vi "Intensity Measurement 2.0.vi"() -> ()   [LabVIEW 2012]
uses:
  <vilib>/Analysis/NI_AAL_SigProc.lvlib
  <vilib>/Analysis/NI_AALBase.lvlib
  <userlib>/_OpenG.lib/array/array.llb/Index 1D Array Elements (DBL)__ogtk.vi
  <vilib>/Analysis/baseanly.llb/Mean (DBL).vi
  Intensity Data.ctl
  <vilib>/Utility/file.llb/Read From Spreadsheet File (I64).vi
  <vilib>/Utility/miscctls.llb/LVPointTypeDef.ctl
  <userlib>/_OpenG.lib/array/array.llb/Conditional Auto-Indexing Tunnel (DBL)__ogtk.vi
  <userlib>/_OpenG.lib/array/array.llb/Conditional Auto-Indexing Tunnel (U32)__ogtk.vi
  <userlib>/_OpenG.lib/array/array.llb/Index 1D Array Elements (U32)__ogtk.vi
  <vilib>/Analysis/6fits.llb/Curve Fitting Criteria.ctl
  <vilib>/Analysis/NI_AALPro.lvlib
panel:
  in  "Tab Control":enum32{"Normalization", "Fitting", "Statistics"}(tab)
  out "Normalization Curve":dbl[](graph)
  out "Normalization Selections":cluster{i32[], i32[]}(graph)
  in  "Reset Normalization Cursors":bool
  in  "Array Type":bool=TRUE
  in  "Load New Data":bool
  in  "pixels/um":dbl=1.0
  in  "Previous Cell":bool
  in  "Next Cell":bool
  in  "Gaussian Fit Method":T1 items=["Least Square", "Least Absolute Residual", "Bisquare"]
  out "Normalized Intensity Maximums":T2(graph)
  out "FWHM":dbl
  out "center":dbl
  out "residue":dbl
  out "amplitude":dbl
  out "Selected Frame":dbl
  out "Peak Fitting":cluster{"Locations":dbl[], "Amplitudes":dbl[]}[](graph)
  in  "Intensity Threshold":i32=50
  out "Cells Identified":i32
  in  "Padding":u32=3
  in  "Target Baseline (%)":dbl=10.0
  out "Cell Width Histogram":T3(graph)
  in  "location histogram interval":i32=10 caption="histogram interval"
  out "Cell Location histogram":T3(graph)
  in  "Gate Width":u32=8 caption="um"
  in  "Gate Center":u32=10 caption="um"
  out "% population\nin gate":dbl
  in  "find best gate center":bool
  out "Arrival time delta histogram":T3(graph)
  in  "Frame Rate":u32=1 min=1 step=1
  in  "arrival histogram interval":i32=10 caption="histogram interval"
  in  "delta threshold":dbl min=0.0
  out "Cell Count":i32
  in  "cell width histo intervals":i32=10 caption="histogram interval"
  # "Cell Selector"
  # "Gaussian Fit"
  # "Statistics"
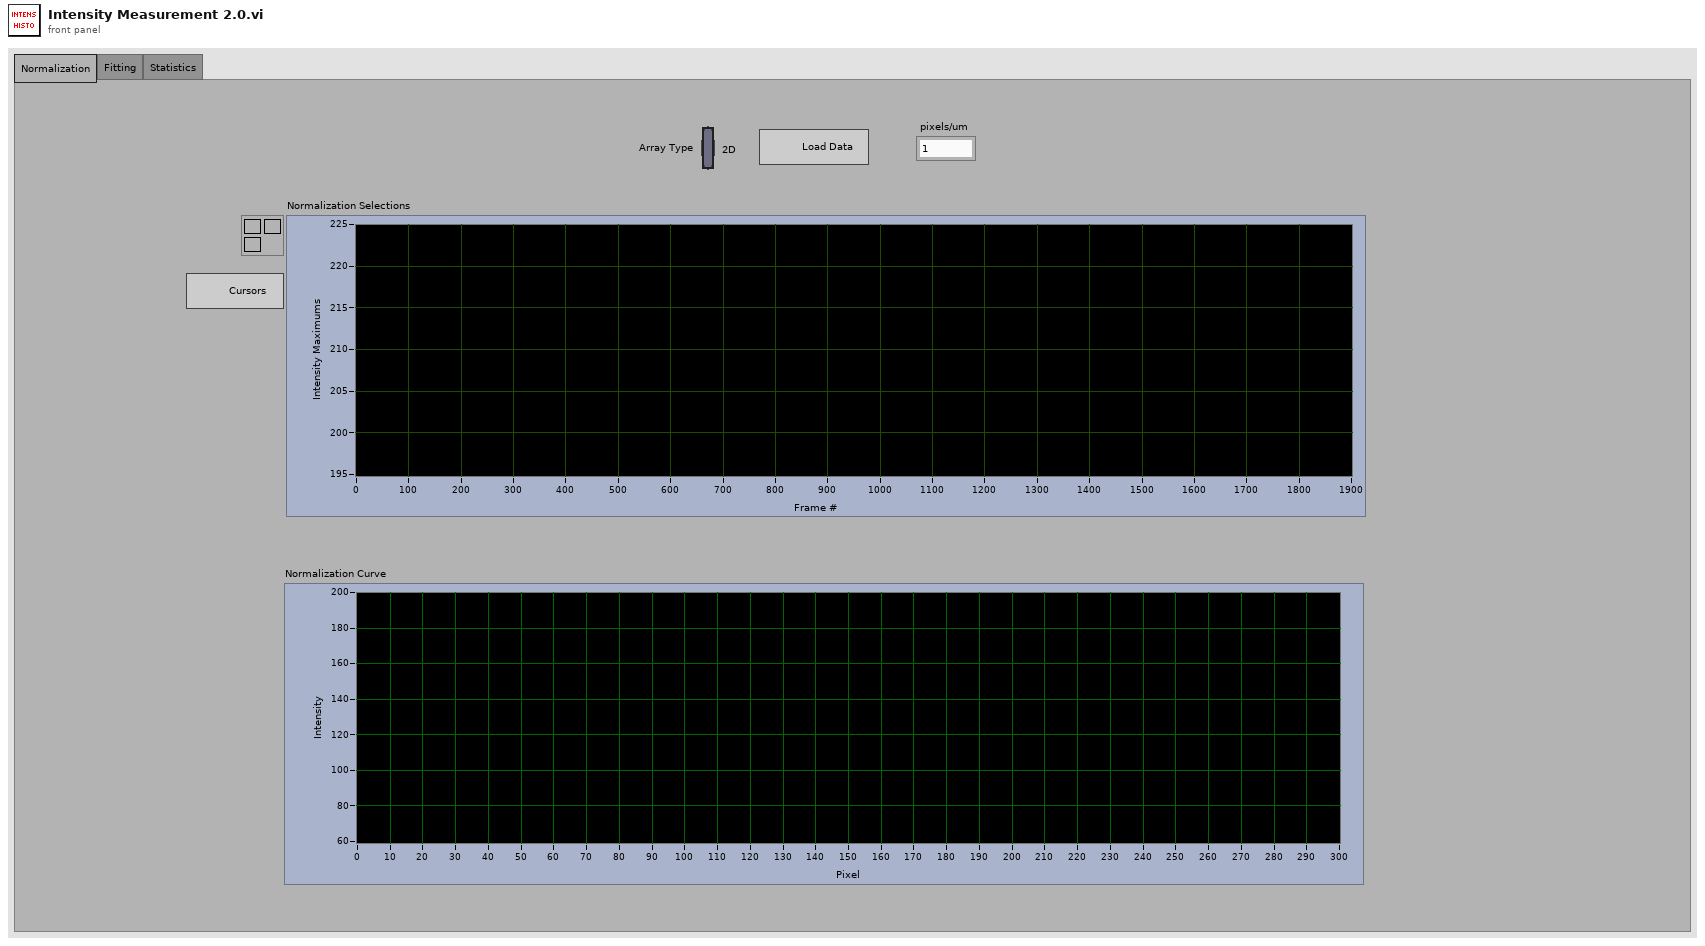
[diagram p1: front panel]
types:
  T1 = typedef "NI_AALPro.lvlib/Curve Fitting Criteria.ctl" = u16
  T2 = cluster{"Cell Location (frame)":u32[], "Cell Amplitude":dbl[]}[]
  T3 = cluster{"X Values":dbl[], "Histogram: h(x)":i32[]}
  T4 = enum32{"invalid app kind", "Development System", "Run Time System", "Student Edition", "Embedded LabVIEW", "Evaluation", "Custom"}
  T5 = cluster{"peak location (frame)":u32[], "Peak Amplitude":dbl[]}[]
  T6 = typedef "LVPointTypeDef.ctl" = cluster{"Horizontal":i16, "Vertical":i16}
  T7 = enum32{"Invalid", "Standard", "Closed", "Hidden", "Minimized", "Maximized"}
  T8 = typedef "Intensity Data.ctl" = cluster{"Raw Data":i32[][], "Normalized Intensity Data":dbl[][], "Frame Count":u32, "Pixel Count":u32, "Interrogation Width (um)":dbl, "Fitting Range":u32[], "Frame Indexed":cluster{"intensity peak":dbl[], "peak location (um)":dbl[]}, "Cell Indexed":cluster{"Cell Location (frame)":u32[], "Cell Amplitude":dbl[], "Cell Location (um)":dbl[], "Cell Width (um)":dbl[], "Cell Arrival Delta (frame)":dbl[], "Cell Arrival Delta (us)":dbl[]}}
  T9 = cluster{"Core":cluster{"Current VI Reference":refnum<vi>, "Close Panel on Exit?":bool}, "Intensity Data Location":path, "pixels/um":dbl, "Intensity Data":T8, "Gated Data":cluster{"Gate Width":u32, "Gate Center":u32, "Cell Indexed":cluster{"Peak Amplitude":dbl[], "peak location (frame)":u32[], "peak location (um)":dbl[]}}}
  T10 = typedef "LVRangeTypeDef.ctl" = cluster{"Minimum":dbl, "Maximum":dbl, "Increment":dbl, "Minor Increment":dbl, "Start":dbl}
  T11 = typedef "LVCursorListTypeDef.ctl" = cluster{"Name":string, "Color":u32, "Style":u8, "Point Style":u8, "Name Visible":bool, "Allow Drag":bool, "Cursor Mode":u32, "Plot":i32, "Index":i32, "Position":cluster{"X":dbl, "Y":dbl}, "X Scale":u32, "Y Scale":u32, "Watch Plots":i32[], "Watch All Plots":bool, "Plot Area":i32, "Label Offset":cluster{"X":dbl, "Y":dbl}}[]
  T12 = cluster{"Name":string, "Color":u32, "Style":u8, "Point Style":u8, "Name Visible":bool, "Allow Drag":bool, "Cursor Mode":u32, "Plot":i32, "Index":i32, "Position":cluster{"X":dbl, "Y":dbl}, "X Scale":u32, "Y Scale":u32, "Watch Plots":i32[], "Watch All Plots":bool, "Plot Area":i32, "Label Offset":cluster{"X":dbl, "Y":dbl}}
  T13 = cluster{"Name":string, "Color":u32, "Style":u8, "Point Style":u8, "Name Visible":bool, "Allow Drag":bool, "Cursor Mode":u32, "Plot":i32, "Index":i32, "Position":cluster{"X":dbl, "Y":dbl}, "X Scale":u32, "Y Scale":u32, "Watch Plots":i32[], "Watch All Plots":bool, "Plot Area":i32, "Label Offset":cluster{"X":dbl, "Y":dbl}}[]
  T14 = cluster{"Gate Width":u32, "Gate Center":u32, "Cell Indexed":cluster{"Peak Amplitude":dbl[], "peak location (frame)":u32[], "peak location (um)":dbl[]}}
  T15 = cluster{"Current VI Reference":refnum<vi>, "Close Panel on Exit?":bool}
  T16 = cluster{"amplitude":dbl, "center":dbl, "FWHM":dbl, "residue":dbl, "Best Gaussian Fit":dbl[]}
  T17 = cluster{"Cell Location (frame)":u32[], "Cell Amplitude":dbl[]}
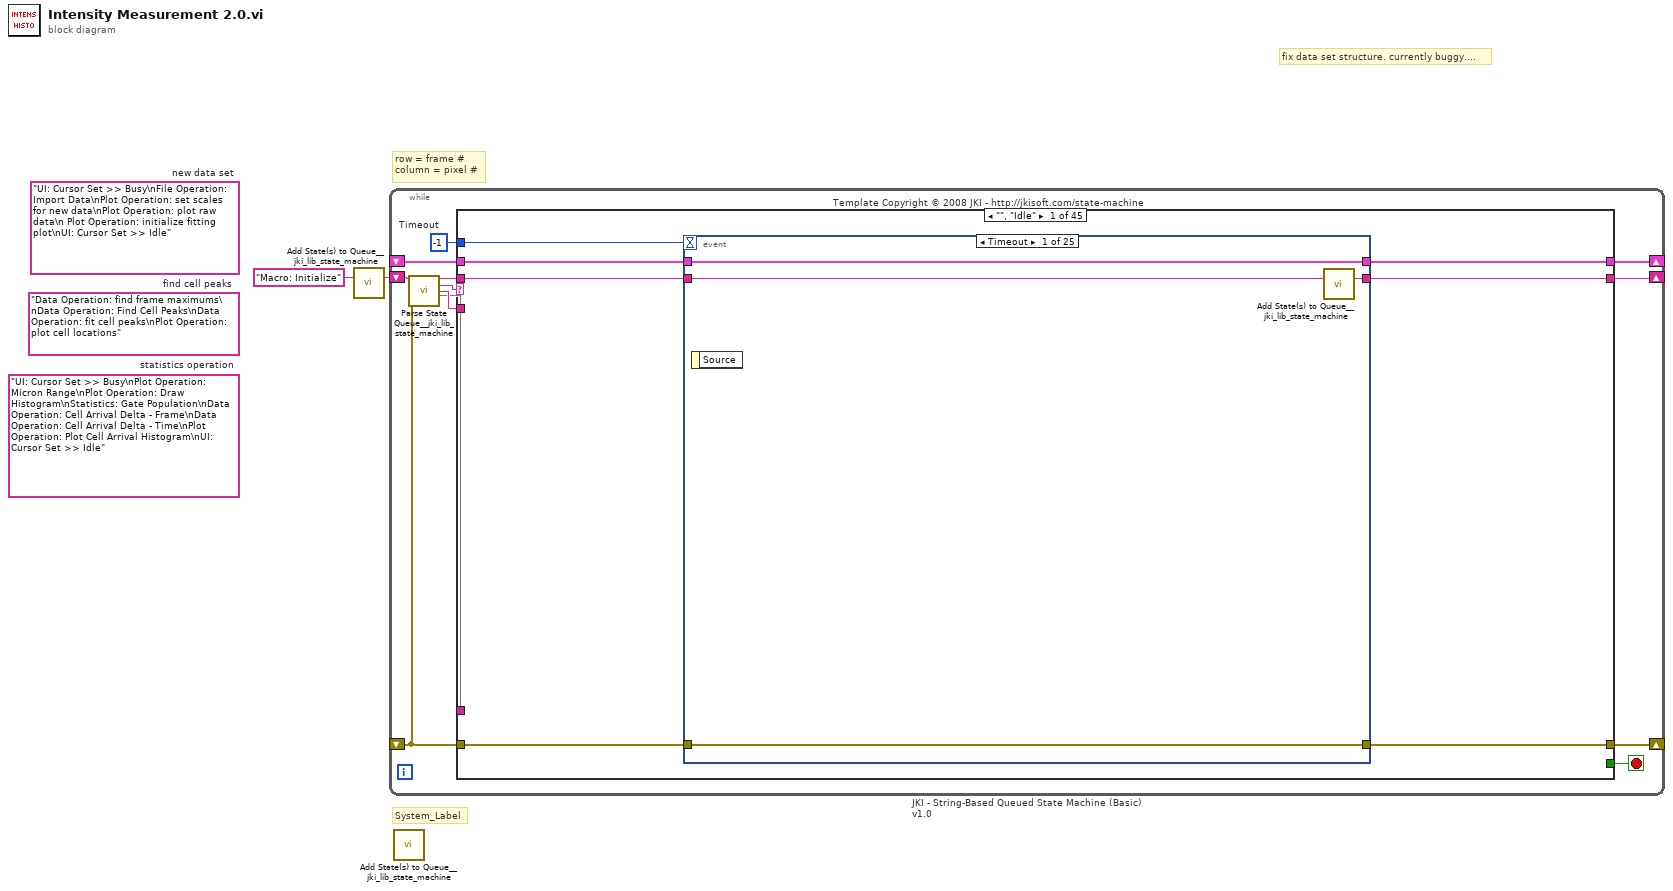
[diagram p0: block diagram]
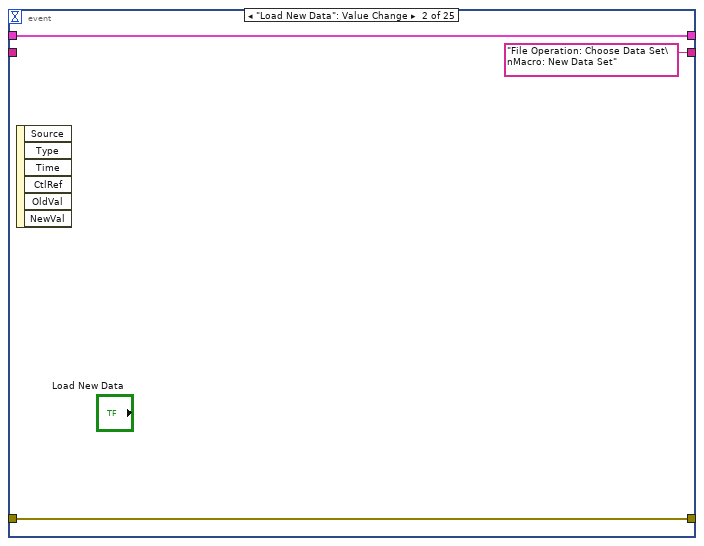
[diagram p2: hidden frame]
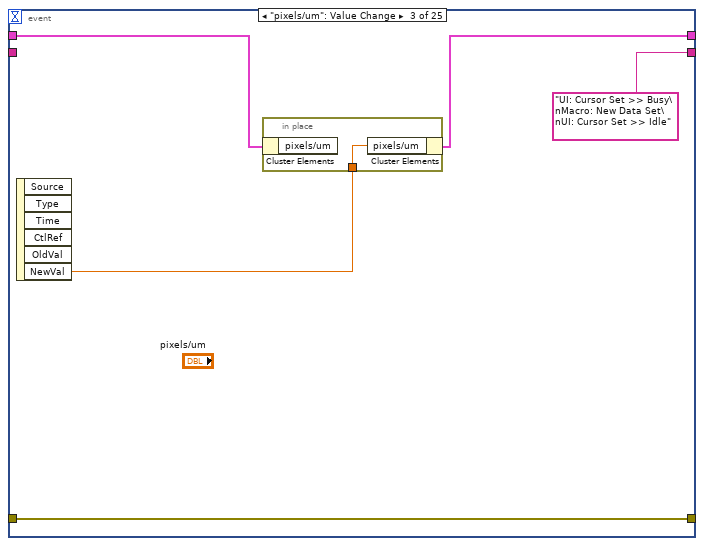
[diagram p3: hidden frame]
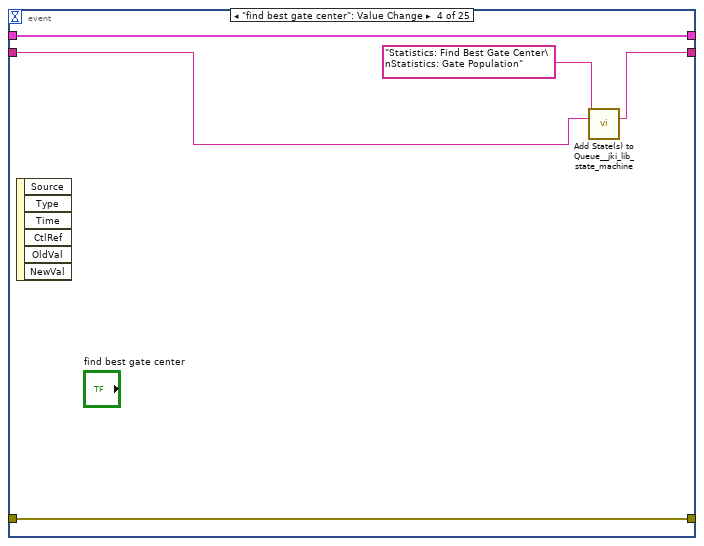
[diagram p4: hidden frame]
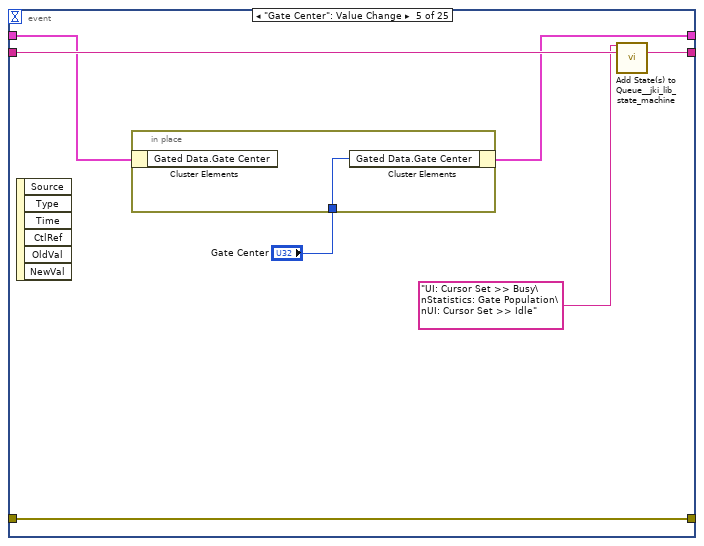
[diagram p5: hidden frame]
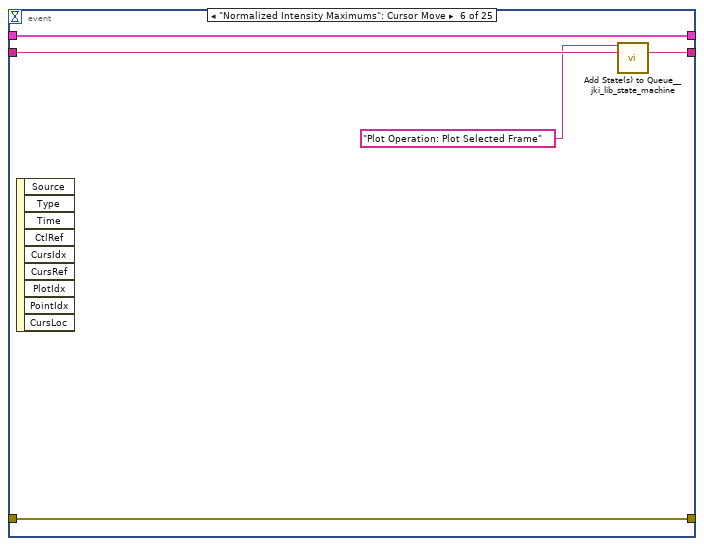
[diagram p6: hidden frame]
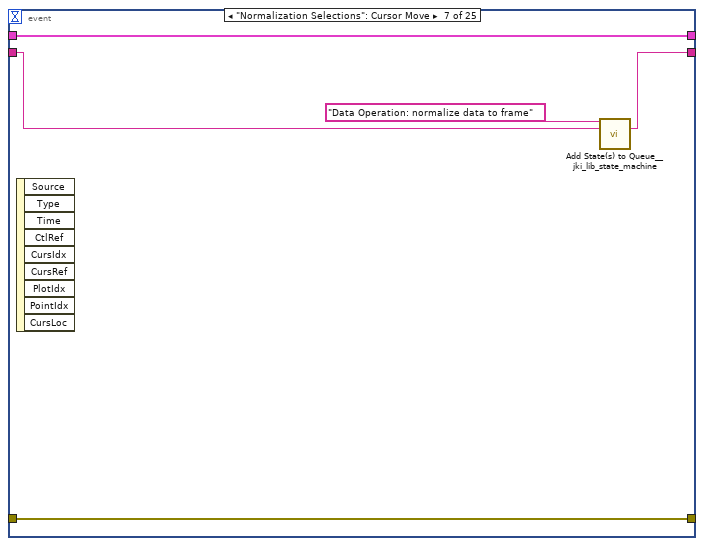
[diagram p7: hidden frame]
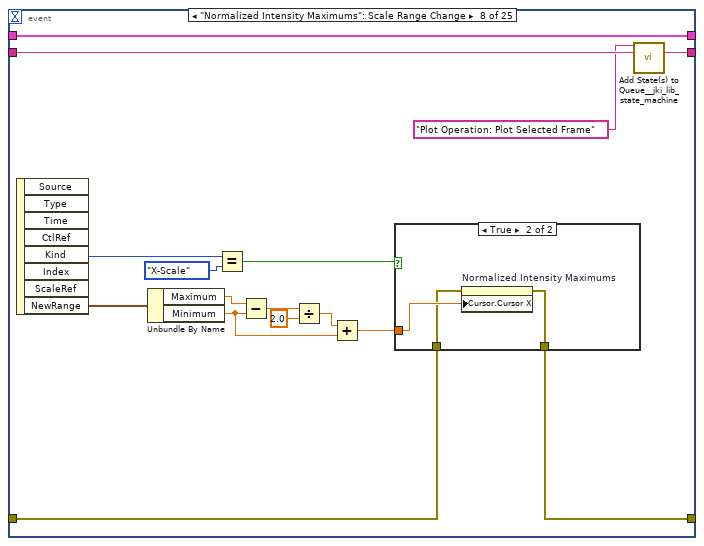
[diagram p8: hidden frame]
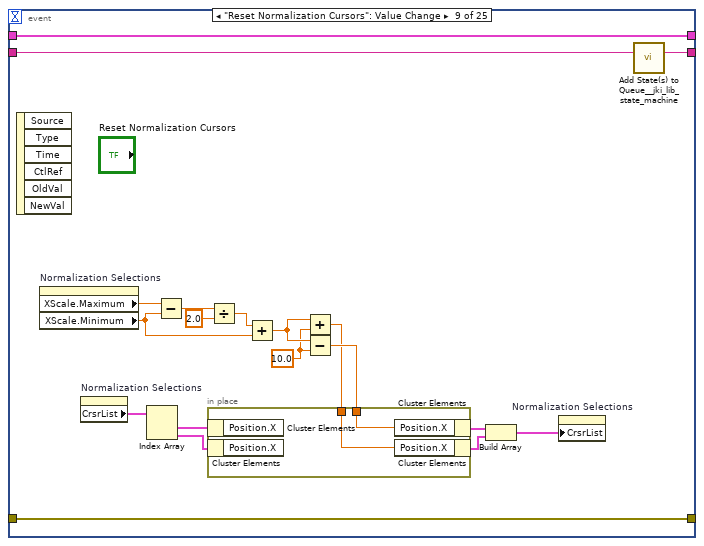
[diagram p10: hidden frame]
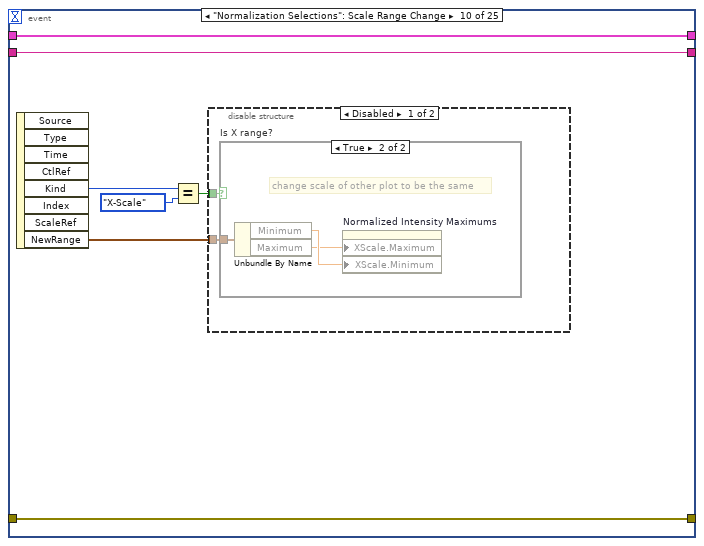
[diagram p11: hidden frame]
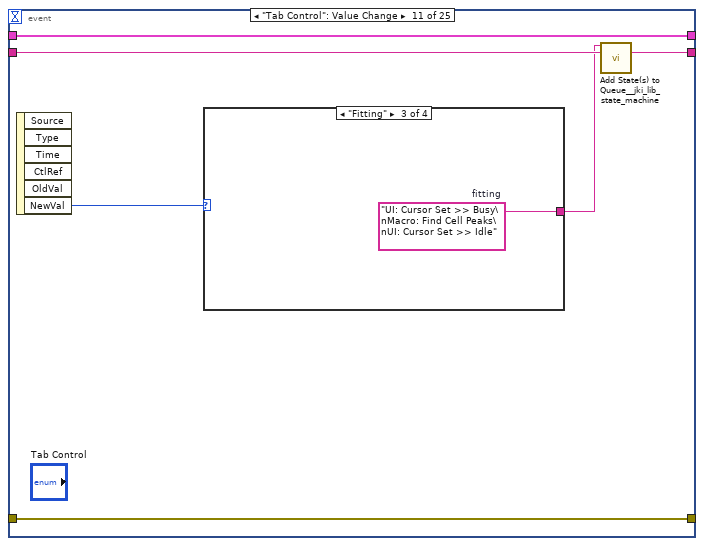
[diagram p14: hidden frame]
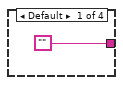
[diagram p15: hidden frame]
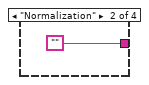
[diagram p16: hidden frame]
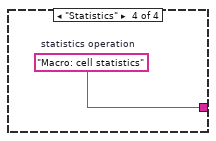
[diagram p17: hidden frame]
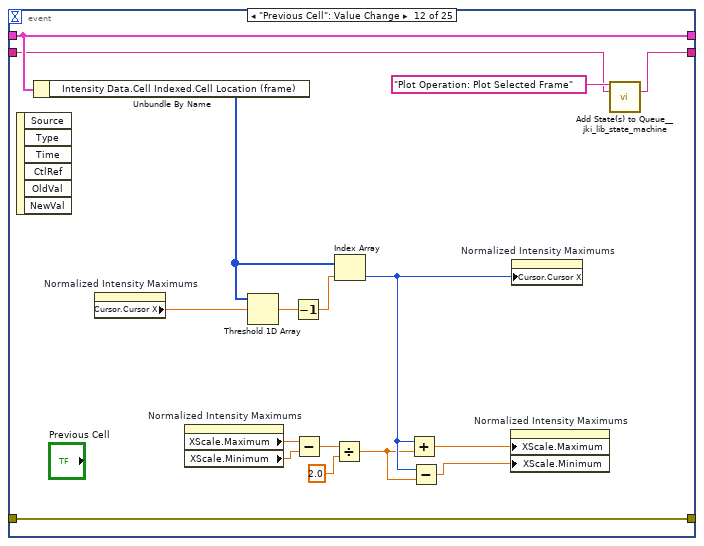
[diagram p18: hidden frame]
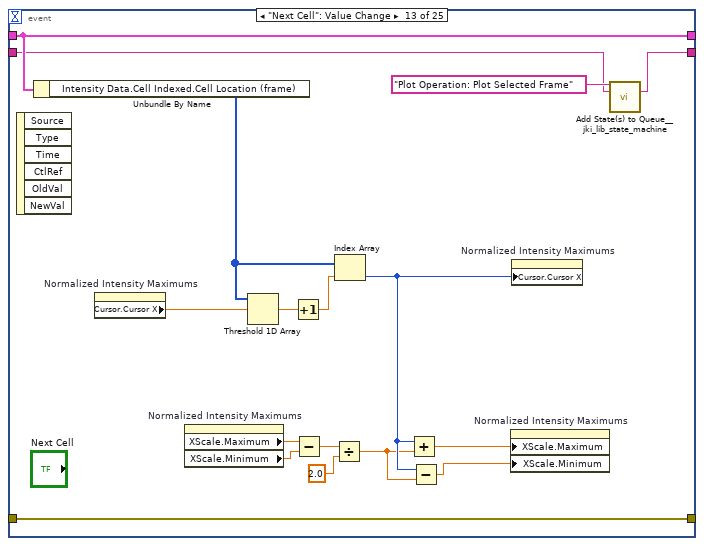
[diagram p19: hidden frame]
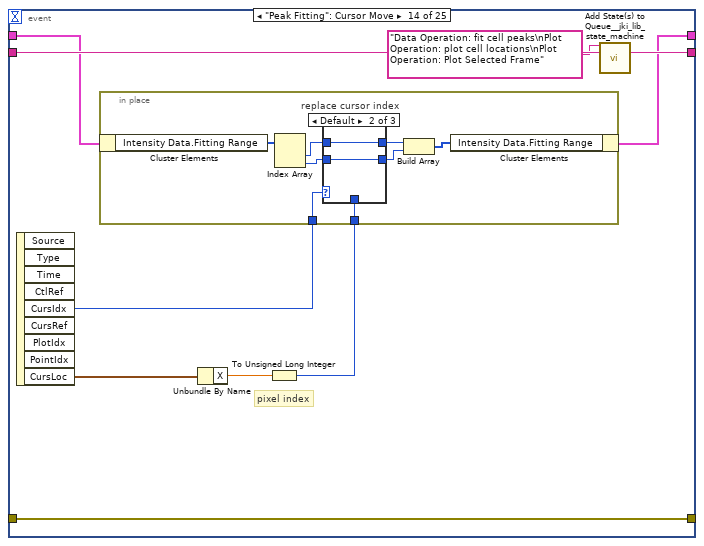
[diagram p20: hidden frame]
diagram:
  (unwired) "UI: Cursor Set >> Busy\nFile Operation: Import Data\nPlot Operation: set scales for new data\nPlot Operation: plot raw data\n Plot Operation: initialize fitting plot\nUI: Cursor Set >> Idle"  # new data set
  (unwired) "Data Operation: find frame maximums\nData Operation: Find Cell Peaks\nData Operation: fit cell peaks\nPlot Operation: plot cell locations"  # find cell peaks
  (unwired) "UI: Cursor Set >> Busy\nPlot Operation: Micron Range\nPlot Operation: Draw Histogram\nStatistics: Gate Population\nData Operation: Cell Arrival Delta - Frame\nData Operation: Cell Arrival Delta - Time\nPlot Operation: Plot Cell Arrival Histogram\nUI: Cursor Set >> Idle"  # statistics operation
  # "fix data set structure. currently buggy...."
  # "row = frame #\ncolumn = pixel #"
  # "System_Label"
  n1 = call <vilib>:"Add State(s) to Queue__jki_lib_state_machine.vi"("State(s) in (\"\")"="Macro: Initialize") -> ("States Out"=w2:string)  [unwired: 14 in]
  n2 = while "JKI - String-Based Queued State Machine (Basic) v1.0" {
    shift-right: [w7] -> _
    shift-left: _ -> [w6]
    shift-right: [w10] -> _
    shift-left: _ -> [w4]
    shift-right: [w9] -> _
    shift-left: w2 -> [w11]
    stop <- w8 stop-if-true
    w5 = -1  # Timeout
    # "Template Copyright © 2008 JKI - http://jkisoft.com/state-machine"
    n3 = call <vilib>:"Parse State Queue__jki_lib_state_machine.vi"("State Queue"=w11, "Error In (no error)"=w4) -> ("Remaining States"=w13:string, "Current State"=w14:string, "Arguments"=w12:string, 14:w3)  [unwired: 10 in]
    n4 = case shown="\"\", \"Idle\"" w14 {
      selector: w14 -> [_ _ w240 _ _ _ _ _ _ _ _ _ _ _ _ _ _ _ _ _ _ _ _ _ _ _ _ _ _ _ _ _ _ _ _ _ _ _ _ _ _ _ _ _ _]
      tunnel: w13 -> [w21 w239 w244 w262 _ w277 w281 w293 w299 w303 w314 w333 w339 w350 w376 w381 w386 w391 w396 w406 w410 w428 w451 w471 w486 w515 w542 w553 w573 w578 w585 w595 w615 w631 w647 w663 w681 w692 w701 w706 w726 w742 w751 w757 w790]
      tunnel: w12 -> [_ _ _ _ _ _ _ _ _ _ _ _ w334 w344 _ _ _ _ _ _ _ _ _ _ _ _ _ _ _ _ _ _ _ _ _ _ _ _ _ _ _ _ _ _ _]
      tunnel: w6 -> [w19 w236 w242 w253 w267 w275 w278 _ w294 w300 w311 w322 w337 w346 w373 w378 w383 w388 w393 w403 w407 w425 w446 w468 w482 w512 w539 w548 w567 w575 w582 w597 w612 w629 w636 w661 w679 w688 w698 w703 w724 w732 w748 w759 w785]
      tunnel: [w18 w237 w246 w259 errorcluster {"status"=FALSE, "code"=0, "source"=""} ("error out") w274 w279 w290 w295 w301 w312 w325 w335 w347 w374 w379 w384 w389 w394 w404 w408 w429 w447 w465 w478 w506 w540 w551 w571 w576 w583 w593 w613 w621 w645 w656 w667 w685 w694 w704 w711 w740 w749 w760 w786] -> w10
      tunnel: w4 -> [w17 w237 w245 w259 w265 w274 w279 w290 w296 w301 w312 w324 w336 w348 w374 w379 w384 w389 w394 w404 w408 w420 w448 w465 w480 w507 w540 w551 w571 w576 w583 w596 w613 w621 w645 w657 w678 w686 w702 w704 w712 w740 w749 w761 w787]
      tunnel: [w20 w238 w243 w261 "UI: Cursor Set >> Idle" ("States Out") w276 w280 w292 w298 w302 w313 w332 w338 w349 w375 w380 w385 w390 w395 w405 w409 w427 w450 w470 w485 w514 w541 w552 w572 w577 w584 w594 w614 w630 w646 w662 w680 w691 w700 w705 w725 w741 w750 w756 w789] -> w9
      tunnel: [_ _ _ _ _ TRUE _ _ _ _ _ _ _ _ _ _ _ _ _ _ _ _ _ _ _ _ _ _ _ _ _ _ _ _ _ _ _ _ _ _ _ _ _ _ _] -> w8
      tunnel: [w16 w236 w242 w260 w267 w275 w278 w291 w294 w300 w311 w322 w337 w346 w373 w378 w383 w388 w393 w403 w407 w426 w445 w467 w479 w510 w538 w547 w566 w575 w582 w597 w612 w629 w637 w661 w679 w688 w698 w703 w723 w731 w748 w758 w784] -> w7
      tunnel: w5 -> [w15 _ _ _ _ _ _ _ _ _ _ _ _ _ _ _ _ _ _ _ _ _ _ _ _ _ _ _ _ _ _ _ _ _ _ _ _ _ _ _ _ _ _ _ _]
      tunnel: w3 -> [_ _ _ _ w263 _ _ _ _ _ _ _ _ _ _ _ _ _ _ _ _ _ _ _ _ _ _ _ _ _ _ _ _ _ _ _ _ _ _ _ _ _ _ _ _]
      frame "", "Idle" {
        n5 = event shown="[0] Timeout" {
          selector: _ -> [_ _ _ _ _ _ _ _ _ _ _ _ _ _ _ _ _ _ _ _ _ _ _ _ _]
          dyn-events: _ -> [_ _ _ _ _ _ _ _ _ _ _ _ _ _ _ _ _ _ _ _ _ _ _ _ _]
          timeout: w15 -> [_ _ _ _ _ _ _ _ _ _ _ _ _ _ _ _ _ _ _ _ _ _ _ _ _]
          tunnel: w21 -> [w25 _ _ w35 w44 w49 w55 w59 w91 w103 w113 w130 w147 w162 w180 w188 _ w197 w201 w206 w212 w216 w222 w225 w235]
          tunnel: [w24 "File Operation: Choose Data Set\nMacro: New Data Set" ("States Out") "UI: Cursor Set >> Busy\nMacro: New Data Set\nUI: Cursor Set >> Idle" ("States Out") w37 w45 w50 w53 w60 w92 w103 w112 w129 w146 w161 w179 w189 "UI: Cursor Set >> Busy\nPlot Operation: Draw Histogram\nUI: Cursor Set >> Idle" ("States Out") w196 w200 w207 w211 w215 w220 w226 w234] -> w20
          tunnel: w19 -> [w22 w28 w31 w38 w42 w51 w56 w73 w96 w104 w115 w136 w153 w160 w182 w186 w193 w198 w203 w208 w213 w218 w223 w228 w232]
          tunnel: [w23 w26 w32 w39 w46 w52 w57 w64 w85 w105 w116 w137 w154 w164 w183 w190 w194 w199 w204 w209 w214 w219 w224 w229 w233] -> w18
          tunnel: w17 -> [w23 w26 w32 w39 w46 w52 w57 w65 w85 w105 w116 w137 w154 w164 w183 w190 w194 w199 w204 w209 w214 w219 w224 w229 w233]
          tunnel: [w22 w28 w29 w38 w40 w51 w56 w73 w96 w104 w115 w136 w153 w159 w182 w185 w193 w198 w203 w208 w213 w218 w223 w228 w232] -> w16
          event Timeout {
            n6 = event-data() -> ()  [unwired: 1 in, 1 out]
            n7 = call <vilib>:"Add State(s) to Queue__jki_lib_state_machine.vi"("State(s) in (\"\")"=w25) -> ("States Out"=w24:string)  [unwired: 14 in]
          }
          event "Load New Data": Value Change {
            n8 = event-data() -> ()  [unwired: 1 in, 6 out]
          }
          event "pixels/um": Value Change {
            n9 = event-data() -> ("NewVal"=w30:dbl)  [unwired: 1 in, 5 out]
            n10 = in-place {
              in-place-border: w30 -> [w34]
              n11 = in-place-cluster #1(w31) -> ()  [unwired: 1 out]
              n12 = in-place-cluster #1("pixels/um"=w34) -> (w29:T9)
            }
          }
          event "find best gate center": Value Change {
            n13 = event-data() -> ()  [unwired: 1 in, 6 out]
            n14 = call <vilib>:"Add State(s) to Queue__jki_lib_state_machine.vi"("State(s) in Front (\"\")"="Statistics: Find Best Gate Center\nStatistics: Gate Population" ("State(s) in Front (\"\")"), "State(s) in (\"\")"=w35) -> ("States Out"=w37:string)  [unwired: 13 in]
          }
          event "Gate Center": Value Change {
            n15 = event-data() -> ()  [unwired: 1 in, 6 out]
            n16 = in-place {
              in-place-border: "Gate Center" -> [w47]
              n17 = in-place-cluster #2(w42) -> ()  [unwired: 1 out]
              n18 = in-place-cluster #2("Gated Data.Gate Center"=w47) -> (w40:T9)
            }
            n19 = call <vilib>:"Add State(s) to Queue__jki_lib_state_machine.vi"("State(s) in Front (\"\")"="UI: Cursor Set >> Busy\nStatistics: Gate Population\nUI: Cursor Set >> Idle" ("State(s) in Front (\"\")"), "State(s) in (\"\")"=w44) -> ("States Out"=w45:string)  [unwired: 13 in]
          }
          event "Normalized Intensity Maximums": Cursor Move {
            n20 = event-data() -> ()  [unwired: 1 in, 9 out]
            n21 = call <vilib>:"Add State(s) to Queue__jki_lib_state_machine.vi"("State(s) in Front (\"\")"="Plot Operation: Plot Selected Frame" ("State(s) in Front (\"\")"), "State(s) in (\"\")"=w49) -> ("States Out"=w50:string)  [unwired: 13 in]
          }
          event "Normalization Selections": Cursor Move {
            n22 = event-data() -> ()  [unwired: 1 in, 9 out]
            n23 = call <vilib>:"Add State(s) to Queue__jki_lib_state_machine.vi"("State(s) in Front (\"\")"="Data Operation: normalize data to frame" ("State(s) in Front (\"\")"), "State(s) in (\"\")"=w55) -> ("States Out"=w53:string)  [unwired: 13 in]
          }
          event "Normalized Intensity Maximums": Scale Range Change {
            n24 = event-data() -> ("Kind"=w72:enum16{"X-Scale", "Y-Scale", "Z-Scale"}, "NewRange"=w69:T10)  [unwired: 1 in, 6 out]
            n25 = Unbundle By Name(w69) -> ("Maximum"=w68:dbl, "Minimum"=w62:dbl)
            n26 = Equal?(x=w72, y=enum16{"X-Scale", "Y-Scale", "Z-Scale"}."X-Scale" ("Kind")) -> (x = y?=w70:bool)
            n27 = Subtract(x=w68, y=w62) -> (x-y=w67:dbl)
            n28 = Divide(x=w67, y=2.0) -> (x/y=w63:dbl)
            n29 = Add(x=w63, y=w62) -> (x+y=w61:dbl)
            n30 = case shown="True" w70 {
              tunnel: w61 -> [_ w77]
              tunnel: w65 -> [w74 w76]
              tunnel: [w74 w75] -> w64
              frame False {
              }
              frame True {
                n31 = property on="Normalized Intensity Maximums" class="XYGraph (strict)"(error in=w76, "Cursor.Cursor X"=w77) -> (error out=w75:errorcluster)  [unwired: 1 in, 1 out]
              }
            }
            n32 = call <vilib>:"Add State(s) to Queue__jki_lib_state_machine.vi"("State(s) in Front (\"\")"="Plot Operation: Plot Selected Frame" ("State(s) in Front (\"\")"), "State(s) in (\"\")"=w59) -> ("States Out"=w60:string)  [unwired: 13 in]
          }
          event "Reset Normalization Cursors": Value Change {
            w83 = 10.0 ("y")
            n33 = event-data() -> ()  [unwired: 1 in, 6 out]
            n34 = property on="Normalization Selections" class="XYGraph (strict)"() -> ("XScale.Maximum"=w87:dbl, "XScale.Minimum"=w86:dbl)  [unwired: 2 in, 2 out]
            n35 = property on="Normalization Selections" class="XYGraph (strict)"() -> ("CrsrList"=w90:T11)  [unwired: 2 in, 2 out]
            n36 = Index Array(array=w90) -> (element #1=w89:T12, element #2=w88:T12)  [unwired: 2 in]
            n37 = Subtract(x=w87, y=w86) -> (x-y=w95:dbl)
            n38 = Divide(x=w95, y=2.0) -> (x/y=w93:dbl)
            n39 = Add(x=w93, y=w86) -> (x+y=w84:dbl)
            n40 = Add(x=w84, y=w83) -> (x+y=w81:dbl)
            n41 = Subtract(x=w84, y=w83) -> (x-y=w82:dbl)
            n42 = in-place {
              in-place-border: w82 -> [w98]
              in-place-border: w81 -> [w97]
              n43 = in-place-cluster #3(w89) -> ()  [unwired: 1 out]
              n44 = in-place-cluster #4(w88) -> ()  [unwired: 1 out]
              n45 = in-place-cluster #3("Position.X"=w98) -> (w80:T12)
              n46 = in-place-cluster #4("Position.X"=w97) -> (w79:T12)
            }
            n47 = Build Array(w80, w79) -> (w78:T13)
            n48 = property on="Normalization Selections" class="XYGraph (strict)"("CrsrList"=w78) -> ()  [unwired: 2 in, 2 out]
            n49 = call <vilib>:"Add State(s) to Queue__jki_lib_state_machine.vi"("State(s) in (\"\")"=w91) -> ("States Out"=w92:string)  [unwired: 14 in]
          }
          event "Normalization Selections": Scale Range Change {
            n50 = event-data() -> ("Kind"=w100:enum16{"X-Scale", "Y-Scale", "Z-Scale"}, "NewRange"=w102:T10)  [unwired: 1 in, 6 out]
            n51 = Equal?(x=w100, y=enum16{"X-Scale", "Y-Scale", "Z-Scale"}."X-Scale" ("Kind")) -> (x = y?=w99:bool)
            n52 = disable-structure shown="Disabled" {
              disable-tunnel: w102 -> [w107 _]
              disable-tunnel: w99 -> [w106 _]
              frame Disabled {
                n53 = case "Is X range?" shown="True" w106 {
                  tunnel: w107 -> [_ w110]
                  frame False {
                  }
                  frame True {
                    # "change scale of other plot to be the same"
                    n54 = Unbundle By Name(w110) -> ("Minimum"=w109:dbl, "Maximum"=w108:dbl)
                    n55 = property on="Normalized Intensity Maximums" class="XYGraph (strict)"("XScale.Maximum"=w108, "XScale.Minimum"=w109) -> ()  [unwired: 2 in, 2 out]
                  }
                }
              }
              frame Enabled {
              }
            }
          }
          event "Tab Control": Value Change {
            n56 = event-data() -> ("NewVal"=w114:enum32{"Normalization", "Fitting", "Statistics"})  [unwired: 1 in, 5 out]
            n57 = case shown="\"Fitting\"" w114 {
              tunnel: ["" "" w119 w120] -> w111
              frame Default {
              }
              frame "Normalization" {
              }
              frame "Fitting" {
                w119 = "UI: Cursor Set >> Busy\nMacro: Find Cell Peaks\nUI: Cursor Set >> Idle"  # fitting
              }
              frame "Statistics" {
                w120 = "Macro: cell statistics"  # statistics operation
              }
            }
            n58 = call <vilib>:"Add State(s) to Queue__jki_lib_state_machine.vi"("State(s) in Front (\"\")"=w111, "State(s) in (\"\")"=w113) -> ("States Out"=w112:string)  [unwired: 13 in]
          }
          event "Previous Cell": Value Change {
            n59 = event-data() -> ()  [unwired: 1 in, 6 out]
            n60 = Unbundle By Name(w136) -> ("Intensity Data.Cell Indexed.Cell Location (frame)"=w134:u32[])
            n61 = property on="Normalized Intensity Maximums" class="XYGraph (strict)"() -> ("Cursor.Cursor X"=w135:dbl)  [unwired: 2 in, 2 out]
            n62 = property on="Normalized Intensity Maximums" class="XYGraph (strict)"() -> ("XScale.Maximum"=w128:dbl, "XScale.Minimum"=w127:dbl)  [unwired: 2 in, 2 out]
            n63 = Threshold 1D Array(2:w135, 3:w134) -> (0:w133:dbl)  [unwired: 1 in]
            n64 = Decrement(x=w133) -> (x-1=w132:dbl)
            n65 = Subtract(x=w128, y=w127) -> (x-y=w126:dbl)
            n66 = Divide(x=w126, y=2.0) -> (x/y=w123:dbl)
            n67 = Index Array(array=w134, index=w132) -> (element=w124:u32)
            n68 = Add(x=w124, y=w123) -> (x+y=w122:dbl)
            n69 = Subtract(x=w124, y=w123) -> (x-y=w121:dbl)
            n70 = property on="Normalized Intensity Maximums" class="XYGraph (strict)"("XScale.Maximum"=w122, "XScale.Minimum"=w121) -> ()  [unwired: 2 in, 2 out]
            n71 = property on="Normalized Intensity Maximums" class="XYGraph (strict)"("Cursor.Cursor X"=w124) -> ()  [unwired: 2 in, 2 out]
            n72 = call <vilib>:"Add State(s) to Queue__jki_lib_state_machine.vi"("State(s) in Front (\"\")"="Plot Operation: Plot Selected Frame" ("State(s) in Front (\"\")"), "State(s) in (\"\")"=w130) -> ("States Out"=w129:string)  [unwired: 13 in]
          }
          event "Next Cell": Value Change {
            n73 = event-data() -> ()  [unwired: 1 in, 6 out]
            n74 = Unbundle By Name(w153) -> ("Intensity Data.Cell Indexed.Cell Location (frame)"=w151:u32[])
            n75 = property on="Normalized Intensity Maximums" class="XYGraph (strict)"() -> ("Cursor.Cursor X"=w152:dbl)  [unwired: 2 in, 2 out]
            n76 = property on="Normalized Intensity Maximums" class="XYGraph (strict)"() -> ("XScale.Maximum"=w145:dbl, "XScale.Minimum"=w144:dbl)  [unwired: 2 in, 2 out]
            n77 = Threshold 1D Array(2:w152, 3:w151) -> (0:w150:dbl)  [unwired: 1 in]
            n78 = Increment(x=w150) -> (x+1=w149:dbl)
            n79 = Subtract(x=w145, y=w144) -> (x-y=w143:dbl)
            n80 = Divide(x=w143, y=2.0) -> (x/y=w140:dbl)
            n81 = Index Array(array=w151, index=w149) -> (element=w141:u32)
            n82 = Add(x=w141, y=w140) -> (x+y=w139:dbl)
            n83 = Subtract(x=w141, y=w140) -> (x-y=w138:dbl)
            n84 = property on="Normalized Intensity Maximums" class="XYGraph (strict)"("XScale.Maximum"=w139, "XScale.Minimum"=w138) -> ()  [unwired: 2 in, 2 out]
            n85 = property on="Normalized Intensity Maximums" class="XYGraph (strict)"("Cursor.Cursor X"=w141) -> ()  [unwired: 2 in, 2 out]
            n86 = call <vilib>:"Add State(s) to Queue__jki_lib_state_machine.vi"("State(s) in Front (\"\")"="Plot Operation: Plot Selected Frame" ("State(s) in Front (\"\")"), "State(s) in (\"\")"=w147) -> ("States Out"=w146:string)  [unwired: 13 in]
          }
          event "Peak Fitting": Cursor Move {
            # "pixel index"
            n87 = event-data() -> ("CursIdx"=w158:i32, "CursLoc"=w163:cluster{"X":dbl, "Y":dbl})  [unwired: 1 in, 7 out]
            n88 = Unbundle By Name(w163) -> ("X"=w156:dbl)
            n89 = To Unsigned Long Integer(number=w156) -> (unsigned 32bit integer=w157:u32)
            n90 = in-place {
              in-place-border: w158 -> [w172]
              in-place-border: w157 -> [w171]
              n91 = in-place-cluster #5(w160) -> ("Intensity Data.Fitting Range"=w170:u32[])
              n92 = Index Array(array=w170) -> (element #1=w169:u32, element #2=w168:u32)  [unwired: 2 in]
              n93 = case "replace cursor index" shown="Default" w172 {
                tunnel: [w174 w175 w177] -> w166
                tunnel: w168 -> [w174 w175 _]
                tunnel: w169 -> [_ w176 w178]
                tunnel: [w173 w176 w178] -> w167
                tunnel: w171 -> [w173 _ w177]
                frame 0 {
                }
                frame Default {
                }
                frame 1 {
                }
              }
              n94 = Build Array(w167, w166) -> (w165:u32[])
              n95 = in-place-cluster #5("Intensity Data.Fitting Range"=w165) -> (w159:T9)
            }
            n96 = call <vilib>:"Add State(s) to Queue__jki_lib_state_machine.vi"("State(s) in Front (\"\")"="Data Operation: fit cell peaks\nPlot Operation: plot cell locations\nPlot Operation: Plot Selected Frame" ("State(s) in Front (\"\")"), "State(s) in (\"\")"=w162) -> ("States Out"=w161:string)  [unwired: 13 in]
          }
          event Value Change {
            n97 = event-data() -> ()  [unwired: 1 in, 6 out]
            n98 = call <vilib>:"Add State(s) to Queue__jki_lib_state_machine.vi"("State(s) in Front (\"\")"="Plot Operation: Plot Selected Frame" ("State(s) in Front (\"\")"), "State(s) in (\"\")"=w180) -> ("States Out"=w179:string)  [unwired: 13 in]
          }
          event "Gate Width": Value Change {
            n99 = event-data() -> ()  [unwired: 1 in, 6 out]
            n100 = in-place {
              in-place-border: "Gate Width" -> [w191]
              n101 = in-place-cluster #6(w186) -> ()  [unwired: 1 out]
              n102 = in-place-cluster #6("Gated Data.Gate Width"=w191) -> (w185:T9)
            }
            n103 = call <vilib>:"Add State(s) to Queue__jki_lib_state_machine.vi"("State(s) in Front (\"\")"="UI: Cursor Set >> Busy\nStatistics: Gate Population\nUI: Cursor Set >> Idle" ("State(s) in Front (\"\")"), "State(s) in (\"\")"=w188) -> ("States Out"=w189:string)  [unwired: 13 in]
          }
          event "location histogram interval": Value Change {
            # "finish this"
            n104 = event-data() -> ()  [unwired: 1 in, 6 out]
          }
          event "delta threshold": Value Change {
            n105 = event-data() -> ()  [unwired: 1 in, 6 out]
            n106 = call <vilib>:"Add State(s) to Queue__jki_lib_state_machine.vi"("State(s) in Front (\"\")"="Plot Operation: plot cell arrival histogram" ("State(s) in Front (\"\")"), "State(s) in (\"\")"=w197) -> ("States Out"=w196:string)  [unwired: 13 in]
          }
          event "Intensity Threshold": Value Change {
            w202 = "Macro: Find Cell Peaks\nPlot Operation: Plot Selected Frame"  # fitting
            n107 = event-data() -> ()  [unwired: 1 in, 6 out]
            n108 = call <vilib>:"Add State(s) to Queue__jki_lib_state_machine.vi"("State(s) in Front (\"\")"=w202, "State(s) in (\"\")"=w201) -> ("States Out"=w200:string)  [unwired: 13 in]
          }
          event "Padding": Value Change {
            w205 = "Macro: Find Cell Peaks\nPlot Operation: Plot Selected Frame"  # fitting
            n109 = event-data() -> ()  [unwired: 1 in, 6 out]
            n110 = call <vilib>:"Add State(s) to Queue__jki_lib_state_machine.vi"("State(s) in Front (\"\")"=w205, "State(s) in (\"\")"=w206) -> ("States Out"=w207:string)  [unwired: 13 in]
          }
          event "cell width histo intervals": Value Change {
            n111 = event-data() -> ()  [unwired: 1 in, 6 out]
            n112 = call <vilib>:"Add State(s) to Queue__jki_lib_state_machine.vi"("State(s) in Front (\"\")"="Plot Operation: Cell Width Histogram" ("State(s) in Front (\"\")"), "State(s) in (\"\")"=w212) -> ("States Out"=w211:string)  [unwired: 13 in]
          }
          event "Target Baseline (%)": Value Change {
            w217 = "Macro: Find Cell Peaks\nPlot Operation: Plot Selected Frame"  # fitting
            n113 = event-data() -> ()  [unwired: 1 in, 6 out]
            n114 = call <vilib>:"Add State(s) to Queue__jki_lib_state_machine.vi"("State(s) in Front (\"\")"=w217, "State(s) in (\"\")"=w216) -> ("States Out"=w215:string)  [unwired: 13 in]
          }
          event "arrival histogram interval": Value Change {
            n115 = event-data() -> ()  [unwired: 1 in, 6 out]
            n116 = call <vilib>:"Add State(s) to Queue__jki_lib_state_machine.vi"("State(s) in Front (\"\")"="Plot Operation: Plot Cell Arrival Histogram" ("State(s) in Front (\"\")"), "State(s) in (\"\")"=w222) -> ("States Out"=w220:string)  [unwired: 13 in]
          }
          event "Frame Rate": Value Change {
            n117 = event-data() -> ()  [unwired: 1 in, 6 out]
            n118 = call <vilib>:"Add State(s) to Queue__jki_lib_state_machine.vi"("State(s) in Front (\"\")"="Data Operation: Cell Arrival Delta - Time\nPlot Operation: Plot Cell Arrival Histogram" ("State(s) in Front (\"\")"), "State(s) in (\"\")"=w225) -> ("States Out"=w226:string)  [unwired: 13 in]
          }
          event Panel Close? {
            # "Discard the event because we'll close the front panel ourselves in Macro: Exit"
            # "Close Panel button (pressed) Event\n(this executes Macro: Exit to terminate the VI)"
            n119 = event-data() -> ()  [unwired: 1 in, 1 out]
            n120 = event-data("Discard?"=TRUE) -> ()  [unwired: 1 in, 1 out]
            n121 = call <vilib>:"Add State(s) to Queue__jki_lib_state_machine.vi"("State(s) in Front (\"\")"="Macro: Exit", "State(s) in (\"\")"=w235) -> ("States Out"=w234:string)  [unwired: 13 in]
          }
        }
      }
      frame "---------- Core ----------" {
        # "Do not put any code in this frame.\n(it is a separator no-op)"
        n122 = call <vilib>:"Add State(s) to Queue__jki_lib_state_machine.vi"("State(s) in (\"\")"=w239) -> ("States Out"=w238:string)  [unwired: 14 in]
      }
      frame Default {
        w249 = 42 items=["No error", "Argument error", "Memory is full", "Out of zone", "End of file", "File already open", "Generic file I/O error", "File not found", "File permission error", "Disk is full", "Duplicate path", "Too many files open", "System feature not enabled", "Resource file not found", "Cannot add resource", "Resource not found", "Image not found", "Image memory error", "Pen does not exist", "Config type invalid", "Config token not found", "Config parse error", "Config memory error", "Bad external code format", "Bad external code offset", "External code not present", "Null window", "Destroy window error", "Null menu", "Print aborted", "Bad print record", "Print driver error", "Windows error during printing", "Memory error during printing", "Print dialog error", "Generic print error", "Invalid device refnum", "Device not found", "Device parameter error", "Device unit error", "Cannot open device", "Device call aborted", "Generic error", "Cancelled by user", "Object ID too low", "Object ID too high", "Object not in heap", "Unknown heap", "Unknown object (invalid DefProc)", "Unknown object (DefProc not in table)", "Message out of range", "Invalid (null) method", "Unknown message", "Manager call not supported", "Bad address", "Network operation in progress", "Network operation timed out", "Connection is busy", "Network attribute not supported", "Network error", "Address in use", "System out of memory", "Connection aborted", "Connection refused", "Not connected", "Already connected", "Connection closed", "Initialization error (interapplication manager)", "Bad occurrence", "Wait on unbound occurrence handler", "Occurrence queue overflow", "Datalog type conflict", "Unused", "Unrecognized type (interapplication manager)", "Memory corrupt", "Failed to make temporary DLL", "Old CIN version", "Drag socket not found", "Failed to load drop-object", "Failed to register OLE object", "Failed to release OLE object", "Format specifier type mismatch", "Unknown format specifier", "Too few format specifiers", "Too many format specifiers", "Scan failed", "Newer CIN version", "Error converting to variant", "Runtime menu error", "Password tampered", "Variant attribute not found", "Incompatible variant data type", "Event data is not available", "Event Store is not present", "Occurrence is not found", "Event Queue is not created", "Event info is not available", "Refnum passed is NULL", "Error retrieving Class GUID", "Error retrieving CoClass GUID", "Error retrieving TypeLib GUID.", "Bad built application magic bytes.", "Specific driver is different from the specific driver associated with the Logical Name.", "There is no session opened to the class driver.", "Max Error", "MAX - Error with config objects", "MAX - Error loading configuration", "MAX - Group not supported"]
        # "Current State"
        # "Do not delete, rename, or modify this frame.\n(this is used to capture unhandled states and typos)"
        # "Handle mistyped state name (developer tool)"
        n123 = Format Into String(format string="Software Exception: Unhandled State \"%s\"." ("message"), error in=w245, w240) -> (resulting string=w248:string, error out=w247:errorcluster)  [unwired: 1 in]
        n124 = call <vilib>:"Error Cluster From Error Code.vi"("show call chain? (False)"=TRUE, "error in (no error)"=w247, "error message (\"\")"=w248, "error code (0)"=w249) -> ("error out"=w246:errorcluster)  [unwired: 5 in]
        n125 = call <vilib>:"Add State(s) to Queue__jki_lib_state_machine.vi"("State(s) in (\"\")"=w244) -> ("States Out"=w243:string)  [unwired: 14 in]
      }
      frame "Initialize Core Data" {
        # "Do not delete, rename, or modify this frame.\n(this is used to determine panel behavior on exit)"
        # "originally closed?"
        # "exe?"
        # "If panel starts closed or is an EXE, then close it when we exit"
        n126 = property class="VI"() -> ("Front Panel.Open"=w258:bool)  [unwired: 2 in, 2 out]
        n127 = property class="App"() -> ("App.Kind"=w257:T4)  [unwired: 2 in, 2 out]
        n128 = control-ref of="Current VI Reference"() -> (w251:refnum<vi>)
        n129 = Not(x=w258) -> (.not. x?=w255:bool)
        n130 = Equal?(x=w257, y=T4."Run Time System" ("Application:Kind")) -> (x = y?=w254:bool)
        n131 = Or(x=w255, y=w254) -> (x .or. y?=w252:bool)
        n132 = Bundle By Name(cluster=w253, "Core.Current VI Reference"=w251, "Core.Close Panel on Exit?"=w252) -> (w260:T9)
        n133 = call <vilib>:"Add State(s) to Queue__jki_lib_state_machine.vi"("State(s) in (\"\")"=w262) -> ("States Out"=w261:string)  [unwired: 14 in]
      }
      frame "Error Handler" {
        # "Unhandled Error -- Display it"
        # "Handle any errors here.\nYou can also output any states to clean-up after errors occur"
        # "Clear error"
        n134 = in-place "In Place Element Structure" {
          in-place-border: w263 -> [w269]
          n135 = in-place-cluster #7(w265) -> ("source"=w270:string)
          n136 = Format Into String(format string=" (state: %s)" ("initial string"), initial string=w270, w269) -> (resulting string=w272:string)  [unwired: 1 in, 1 out]
          n137 = in-place-cluster #7("source"=w272) -> (w264:errorcluster)
        }
        n138 = call <vilib>:"General Error Handler.vi"("error in (no error)"=w264) -> ()  [unwired: 10 in, 5 out]
      }
      frame "Exit" {
        # "Do not put any code in this frame.\n(No errors that occur here will be handled.)"
        n139 = call <vilib>:"Add State(s) to Queue__jki_lib_state_machine.vi"("State(s) in (\"\")"=w277) -> ("States Out"=w276:string)  [unwired: 14 in]
      }
      frame "---------- Data ----------" {
        # "Do not put any code in this frame.\n(It is a separator no-op. You can make a copy of this frame to create a new Data frame)"
        n140 = call <vilib>:"Add State(s) to Queue__jki_lib_state_machine.vi"("State(s) in (\"\")"=w281) -> ("States Out"=w280:string)  [unwired: 14 in]
      }
      frame "Data: Initialize" {
        w285 = T14 {"Gate Width"=0, "Gate Center"=0, "Cell Indexed"={"Peak Amplitude"=[], "peak location (frame)"=[], "peak location (um)"=[]}}  # Gated Data
        w287 = T8 {"Raw Data"=[], "Normalized Intensity Data"=[], "Frame Count"=0, "Pixel Count"=0, "Interrogation Width (um)"=0.0, "Fitting Range"=[], "Frame Indexed"={"intensity peak"=[], "peak location (um)"=[]}, "Cell Indexed"={"Cell Location (frame)"=[], "Cell Amplitude"=[], "Cell Location (um)"=[], "Cell Width (um)"=[], "Cell Arrival Delta (frame)"=[], "Cell Arrival Delta (us)"=[]}}  # Intensity Data
        w288 = path ""  # Intensity Data Location
        w289 = T15 {"Current VI Reference"=refnum, "Close Panel on Exit?"=FALSE}  # Core
        # "Data names and types of shift register data are defined by this bundle."
        # "Initialize the shift-register data, here.\n(data names are defined by what you wire into the bundle function)"
        n141 = local read "pixels/um"() -> (w286:dbl)
        n142 = local read "Gate Center"() -> (w283:u32)
        n143 = local read "Gate Width"() -> (w282:u32)
        n144 = Bundle By Name(cluster=w285, "Gate Width"=w282, "Gate Center"=w283) -> (w284:T14)
        n145 = Bundle("Core"=w289, "Intensity Data Location"=w288, "pixels/um"=w286, "Intensity Data"=w287, "Gated Data"=w284) -> (w291:T9)  [unwired: 1 in]
        n146 = call <vilib>:"Add State(s) to Queue__jki_lib_state_machine.vi"("State(s) in (\"\")"=w293) -> ("States Out"=w292:string)  [unwired: 14 in]
      }
      frame "Data: Cleanup" {
        # "Cleanup any data and references, here.\n(this is called automatically, by the Macro: Exit)"
        n147 = Unbundle By Name(w294) -> ("Core.Current VI Reference"=w297:refnum<vi>)
        n148 = Close Reference(reference=w297, error in (no error)=w296) -> (error out=w295:errorcluster)
        n149 = call <vilib>:"Add State(s) to Queue__jki_lib_state_machine.vi"("State(s) in (\"\")"=w299) -> ("States Out"=w298:string)  [unwired: 14 in]
      }
      frame "---------- UI ----------" {
        # "Do not put any code in this frame.\n(It is a separator no-op. You can make a copy of this frame to create a new UI frame)"
        n150 = call <vilib>:"Add State(s) to Queue__jki_lib_state_machine.vi"("State(s) in (\"\")"=w303) -> ("States Out"=w302:string)  [unwired: 14 in]
      }
      frame "UI: Initialize Plots" {
        n151 = local write "Arrival time delta histogram"(T3 {"X Values"=[], "Histogram: h(x)"=[]} ("Arrival time delta histogram")) -> ()
        n152 = local write "Cell Width Histogram"(T3 {"X Values"=[], "Histogram: h(x)"=[]} ("Cell Width Histogram")) -> ()
        n153 = local write "Peak Fitting"(cluster{"Locations":dbl[], "Amplitudes":dbl[]}[] [] ("Intensity vs. Pixel location")) -> ()
        n154 = local write "Normalization Selections"(cluster{i32[], i32[]} {[], []} ("Normalization Selections")) -> ()
        n155 = local write "Normalized Intensity Maximums"(T5 [] ("Intensity vs. Frame #")) -> ()
        n156 = local write "Cell Location histogram"(T3 {"X Values"=[], "Histogram: h(x)"=[]} ("Cell Location histogram")) -> ()
        n157 = local write "Normalization Curve"(dbl[] [] ("Normalization Frame")) -> ()
        n158 = call <vilib>:"Add State(s) to Queue__jki_lib_state_machine.vi"("State(s) in (\"\")"=w314) -> ("States Out"=w313:string)  [unwired: 14 in]
      }
      frame "UI: Initialize" {
        # "Initialize the User Interface, here.\n(this is called automatically, by the Macro: Init)"
        n159 = control-ref of="This VI"() -> (w330:refnum<vi>)
        n160 = property class="VI"(reference=w330, error in=w324) -> (reference out=w328:refnum<vi>, error out=w323:errorcluster, "Panel"=w329:refnum<vi>)
        n161 = property class="Pnl"(reference=w329, error in=w323) -> (reference out=w327:refnum<vi>, error out=w319:errorcluster, "Panes[]"=w321:refnum<vi>[])
        n162 = Index Array(array=w321) -> (element=w320:refnum<vi>)  [unwired: 1 in]
        n163 = local write "Tab Control"(enum32{"Normalization", "Fitting", "Statistics"}."Normalization" ("Tab Control")) -> ()
        n164 = property class="Pane"(reference=w320, error in=w319, "Origin"=T6 {"Horizontal"=0, "Vertical"=0}) -> (reference out=w318:refnum<vi>, error out=w317:errorcluster)
        n165 = call <vilib>:"Add State(s) to Queue__jki_lib_state_machine.vi"("State(s) in (\"\")"=w333) -> ("States Out"=w332:string)  [unwired: 14 in]
        n166 = Close Reference(reference=w318, error in (no error)=w317) -> (error out=w316:errorcluster)
        n167 = Close Reference(reference=w327, error in (no error)=w316) -> (error out=w326:errorcluster)
        n168 = Close Reference(reference=w328, error in (no error)=w326) -> (error out=w325:errorcluster)
      }
      frame "UI: Cursor Set" {
        # "Argument"
        # "Set and Unset Cursor Busy.\n(Usage: \"UI: Cursor Set >> Busy|Idle\")"
        n169 = case shown="\"Idle\", Default" w334 {
          tunnel: w336 -> [w341 w343]
          tunnel: [w340 w342] -> w335
          frame "Idle", Default {
            n170 = call <vilib>:"Unset Busy.vi"("error in (no error)"=w341) -> ("error out"=w340:errorcluster)  [unwired: 10 in]
          }
          frame "Busy" {
            n171 = call <vilib>:"Set Busy.vi"("error in (no error)"=w343) -> ("error out"=w342:errorcluster)  [unwired: 9 in, 1 out]
          }
        }
        n172 = call <vilib>:"Add State(s) to Queue__jki_lib_state_machine.vi"("State(s) in (\"\")"=w339) -> ("States Out"=w338:string)  [unwired: 14 in]
      }
      frame "UI: Front Panel State" {
        # "Argument"
        # "Set Front Panel Open or Closed\n(Usage: \"UI: Front Panel State >> Open|Close\")"
        n173 = Unbundle By Name(w346) -> ("Core.Current VI Reference"=w345:refnum<vi>)
        n174 = case shown="\"Open\", Default" w344 {
          tunnel: w348 -> [w354 w367]
          tunnel: [w356 w368] -> w347
          tunnel: w345 -> [w355 w365]
          frame "Open", Default {
            n175 = property class="VI"(reference=w355, error in=w354) -> (reference out=w352:refnum<vi>, error out=w353:errorcluster, "Front Panel.Open"=w351:bool)
            n176 = case shown="False" w351 {
              tunnel: [w359 w362] -> w356
              tunnel: w353 -> [w358 w362]
              tunnel: w352 -> [w357 _]
              frame False {
                n177 = invoke class="VI" method="FP.Open"(reference=w357, error in=w358, "Activate"=TRUE, "State"=T7."Standard") -> (error out=w359:errorcluster)  [unwired: 1 in, 4 out]
              }
              frame True {
              }
            }
          }
          frame "Close" {
            n178 = property class="VI"(reference=w365, error in=w367) -> (reference out=w364:refnum<vi>, error out=w366:errorcluster, "Front Panel.Open"=w363:bool)
            n179 = case shown="True" w363 {
              tunnel: [w369 w372] -> w368
              tunnel: w366 -> [w369 w371]
              tunnel: w364 -> [_ w370]
              frame False {
              }
              frame True {
                n180 = invoke class="VI" method="FP.Close"(reference=w370, error in=w371) -> (error out=w372:errorcluster)  [unwired: 1 in, 2 out]
              }
            }
          }
        }
        n181 = call <vilib>:"Add State(s) to Queue__jki_lib_state_machine.vi"("State(s) in (\"\")"=w350) -> ("States Out"=w349:string)  [unwired: 14 in]
      }
      frame "---------- Macro ----------" {
        # "Do not put any code in this frame.\n(It is a separator no-op. You can make a copy of this frame to create a new Macro frame)"
        n182 = call <vilib>:"Add State(s) to Queue__jki_lib_state_machine.vi"("State(s) in (\"\")"=w376) -> ("States Out"=w375:string)  [unwired: 14 in]
      }
      frame "Macro: New Data Set" {
        w377 = "UI: Cursor Set >> Busy\nFile Operation: Import Data\nPlot Operation: set scales for new data\nPlot Operation: plot raw data\n Plot Operation: initialize fitting plot\nUI: Cursor Set >> Idle"  # new data set
        n183 = call <vilib>:"Add State(s) to Queue__jki_lib_state_machine.vi"("State(s) in Front (\"\")"=w377, "State(s) in (\"\")"=w381) -> ("States Out"=w380:string)  [unwired: 13 in]
      }
      frame "Macro: find cell peaks" {
        w382 = "Data Operation: find frame maximums\nData Operation: Find Cell Peaks\nData Operation: fit cell peaks\nPlot Operation: plot cell locations"  # find cell peaks
        n184 = call <vilib>:"Add State(s) to Queue__jki_lib_state_machine.vi"("State(s) in Front (\"\")"=w382, "State(s) in (\"\")"=w386) -> ("States Out"=w385:string)  [unwired: 13 in]
      }
      frame "Macro: cell statistics" {
        w387 = "UI: Cursor Set >> Busy\nPlot Operation: Micron Range\nPlot Operation: Draw Histogram\nStatistics: Gate Population\nData Operation: Cell Arrival Delta - Frame\nData Operation: Cell Arrival Delta - Time\nPlot Operation: Plot Cell Arrival Histogram\n Plot Operation: Cell Width Histogram\nUI: Cursor Set >> Idle"  # statistics operation
        n185 = call <vilib>:"Add State(s) to Queue__jki_lib_state_machine.vi"("State(s) in Front (\"\")"=w387, "State(s) in (\"\")"=w391) -> ("States Out"=w390:string)  [unwired: 13 in]
      }
      frame "Macro: Initialize" {
        w392 = "Data: Initialize\nInitialize Core Data\nUI: Initialize\nUI: Initialize Plots\nUI: Front Panel State >> Open"  # Data: Initialize Initialize Core Data UI: Initialize UI: Initialize Plots UI: Front Panel State >> Open
        # "Initialization Macro\n(This is called once, when the VI starts)"
        n186 = call <vilib>:"Add State(s) to Queue__jki_lib_state_machine.vi"("State(s) in Front (\"\")"=w392, "State(s) in (\"\")"=w396) -> ("States Out"=w395:string)  [unwired: 13 in]
      }
      frame "Macro: Exit" {
        # "Exit Macro\n(This is called once, when the VI exits)"
        n187 = Unbundle By Name(w403) -> ("Core.Close Panel on Exit?"=w402:bool)
        n188 = Select(t="UI: Front Panel State >> Close", s=w402, f="") -> (s? t:f=w399:string)
        n189 = call <vilib>:"Add State(s) to Queue__jki_lib_state_machine.vi"("State(s) in (\"\")"=w399, "State(s) at Back (\"\")"="Data: Cleanup\nExit") -> ("States Out"=w397:string)  [unwired: 13 in]
        n190 = call <vilib>:"Add State(s) to Queue__jki_lib_state_machine.vi"("State(s) in Front (\"\")"=w397, "State(s) in (\"\")"=w406) -> ("States Out"=w405:string)  [unwired: 13 in]
      }
      frame "---------- Data Operation ----------" {
        # "Template Separator\n(You can make a copy of, or modify, this frame)"
        n191 = call <vilib>:"Add State(s) to Queue__jki_lib_state_machine.vi"("State(s) in (\"\")"=w410) -> ("States Out"=w409:string)  [unwired: 14 in]
      }
      frame "Data Operation: normalize data to frame" {
        # "something wrong with this for loop!!!"
        # "get cursor positions"
        # "Template Separator\n(You can make a copy of, or modify, this frame)"
        n192 = control-ref of="Normalization Selections"() -> (w424:refnum<vi>)
        n193 = property on="Property Node" class="XYGraph (strict)"(reference=w424, error in=w420) -> (error out=w429:errorcluster, "CrsrList"=w423:T11)  [unwired: 1 out]
        n194 = Index Array(array=w423) -> (element #1=w422:T12, element #2=w421:T12)  [unwired: 2 in]
        n195 = Unbundle By Name(w425) -> ("Intensity Data.Raw Data"=w419:i32[][])
        n196 = Unbundle By Name(w422) -> ("Position.X"=w418:dbl)
        n197 = Unbundle By Name(w421) -> ("Position.X"=w417:dbl)
        n198 = call "Create Sorted Range.vi"("b"=w417, "a"=w418) -> ("Sorted Range"=w416:u32[])
        n199 = for "extract frames" {
          tunnel: w419 -> [w437]
          tunnel: w416 -> [w436] mode=indexing
          tunnel: [w435] -> w415 mode=indexing
          tunnel: [w434] -> w414
          n200 = Index Array(array=w437, index (row)=w436) -> (element=w435:i32[])  [unwired: 1 in]
          n201 = Array Size(array=w435) -> (size(s)=w434:i32)
        }
        n202 = for "average pixels" {
          N: w414 -> [_]
          tunnel: w415 -> [w433]
          tunnel: [w430] -> w413 mode=indexing
          i -> [w432]
          n203 = Index Array(array=w433, index (col)=w432) -> (element=w431:i32[])  [unwired: 1 in]
          n204 = call-poly <vilib>:"Mean.vi"("X"=w431) -> ("mean"=w430:dbl)  [unwired: 1 out]
        }
        "Normalization Curve" <- w413
        n205 = for "Normalize Intensity\ndata to referenece pixels" {
          tunnel: w419 -> [w441]
          tunnel: [w440] -> w412 mode=indexing
          tunnel: w413 -> [w442] mode=indexing
          i -> [w438]
          n206 = Index Array(array=w441, index (col)=w438) -> (element=w439:i32[])  [unwired: 1 in]
          n207 = Subtract(x=w439, y=w442) -> (x-y=w440:dbl[])
        }
        n208 = Transpose 2D Array(2D array=w412) -> (transposed array=w411:dbl[][])
        n209 = in-place {
          in-place-border: w411 -> [w443]
          n210 = in-place-cluster #8(w425) -> ()  [unwired: 1 out]
          n211 = in-place-cluster #8("Intensity Data.Normalized Intensity Data"=w443) -> (w426:T9)
        }
        n212 = call <vilib>:"Add State(s) to Queue__jki_lib_state_machine.vi"("State(s) in (\"\")"=w428) -> ("States Out"=w427:string)  [unwired: 14 in]
      }
      frame "Data Operation: Normalize Intensity Data (deprecated)" {
        n213 = Unbundle By Name(w446) -> ("Intensity Data.Raw Data"=w449:i32[][])
        n214 = for "measure SnR in each frame, along with location of peak" {
          shift-right: [w453] -> w447
          shift-left: w448 -> [w460]
          tunnel: w449 -> [w458] mode=indexing
          tunnel: [w457] -> w444 mode=indexing
          stop <- w453 stop-if-true
          # "last value"
          # "first value"
          # "max value"
          n215 = Array Size(array=w458) -> (size(s)=w455:i32)
          n216 = Decrement(x=w455) -> (x-1=w454:i32)
          n217 = Array Max & Min(array=w458) -> (min value=w459:i32)  [unwired: 3 out]
          n218 = Index Array(array=w458) -> (element=w463:i32)  [unwired: 1 in]
          n219 = Index Array(array=w458, index=w454) -> (element=w464:i32)
          n220 = Build Array(w459, w463, w464) -> (w462:i32[])
          n221 = call-poly <vilib>:"Mean.vi"("X"=w462) -> ("mean"=w456:dbl, "error"=w461:i32)
          n222 = Subtract "normalize to baseline"(x=w458, y=w456) -> (x-y=w457:dbl[])
          n223 = call <vilib>:"Error Cluster From Error Code.vi"("error in (no error)"=w460, "error code (0)"=w461) -> ("error out"=w453:errorcluster)  [unwired: 7 in]
        }
        n224 = in-place {
          in-place-border: w444 -> [w452]
          n225 = in-place-cluster #9(w446) -> ()  [unwired: 1 out]
          n226 = in-place-cluster #9("Intensity Data.Normalized Intensity Data"=w452) -> (w445:T9)
        }
        n227 = call <vilib>:"Add State(s) to Queue__jki_lib_state_machine.vi"("State(s) in (\"\")"=w451) -> ("States Out"=w450:string)  [unwired: 14 in]
      }
      frame "Data Operation: find frame maximums" {
        n228 = Unbundle By Name(w468) -> ("Intensity Data.Normalized Intensity Data"=w469:dbl[][])
        n229 = for "measure frame peaks" {
          tunnel: w469 -> [w473] mode=indexing
          tunnel: [w474] -> w466 mode=indexing
          # "peak value"
          n230 = Array Max & Min(array=w473) -> (max value=w474:dbl)  [unwired: 3 out]
        }
        n231 = in-place {
          in-place-border: w466 -> [w472]
          n232 = in-place-cluster #10(w468) -> ()  [unwired: 1 out]
          n233 = in-place-cluster #10("Intensity Data.Frame Indexed.intensity peak"=w472) -> (w467:T9)
        }
        n234 = call <vilib>:"Add State(s) to Queue__jki_lib_state_machine.vi"("State(s) in (\"\")"=w471) -> ("States Out"=w470:string)  [unwired: 14 in]
      }
      frame "Data Operation: Find Cell Peaks" {
        n235 = Unbundle By Name(w482) -> ("Intensity Data.Frame Indexed.intensity peak"=w483:dbl[])
        n236 = local read "Intensity Threshold"() -> (w484:i32)
        n237 = call <vilib>:"Peak Detector.vi"("threshold"=w484, "X"=w483) -> ("error"=w481:i32, "Amplitudes"=w476:dbl[], "Locations"=w475:dbl[], "# found"=→"Cells Identified":i32)  [unwired: 5 in, 1 out]
        n238 = call <vilib>:"Error Cluster From Error Code.vi"("error in (no error)"=w480, "error code (0)"=w481) -> ("error out"=w478:errorcluster)  [unwired: 7 in]
        n239 = in-place {
          in-place-border: w475 -> [w492]
          in-place-border: w478 -> [w490]
          in-place-border: w476 -> [w488]
          n240 = in-place-cluster #11(w482) -> ("Intensity Data.Cell Indexed.Cell Location (frame)"=w491:u32[], "Intensity Data.Cell Indexed.Cell Amplitude"=w487:dbl[])
          n241 = case shown="No Error" w490 {
            tunnel: [w495 w497] -> w493
            tunnel: w492 -> [w495 _]
            tunnel: w491 -> [_ w497]
            tunnel: [w494 w496] -> w489
            tunnel: w488 -> [w494 _]
            tunnel: w487 -> [_ w496]
            frame No Error {
            }
            frame Error {
            }
          }
          n242 = in-place-cluster #11("Intensity Data.Cell Indexed.Cell Location (frame)"=w493, "Intensity Data.Cell Indexed.Cell Amplitude"=w489) -> (w479:T9)
        }
        n243 = call <vilib>:"Add State(s) to Queue__jki_lib_state_machine.vi"("State(s) in (\"\")"=w486) -> ("States Out"=w485:string)  [unwired: 14 in]
      }
      frame "Data Operation: fit cell peaks" {
        # "pixels/um"
        n244 = Unbundle By Name(w512) -> ("pixels/um"=w508:dbl, "Intensity Data.Normalized Intensity Data"=w513:dbl[][], "Intensity Data.Cell Indexed.Cell Location (frame)"=w498:u32[])
        n245 = for "Fit peaks of initial 'cell' locations" {
          tunnel: w513 -> [w534]
          tunnel: w498 -> [w531] mode=indexing
          tunnel: [w530] -> w503 mode=indexing
          tunnel: [w529] -> w505 mode=indexing
          tunnel: [w528] -> w501 mode=indexing
          shift-right: [w526] -> w506
          shift-left: w507 -> [w527]
          tunnel: [w521] -> w499 mode=indexing
          # "valid fit?"
          n246 = local read "Gaussian Fit Method"() -> (w524:T1)
          n247 = local read "Intensity Threshold"() -> (w525:i32)
          n248 = local read "Target Baseline (%)"() -> (w523:dbl)
          n249 = local read "Padding"() -> (w522:u32)
          n250 = Index Array "grab frame"(array=w534, index (row)=w531) -> (element=w532:dbl[])  [unwired: 1 in]
          n251 = call "Find Intensity Peaks V3.vi"("Gaussian Fit Method"=w524, "Padding"=w522, "error in (no error)"=w527, "Target Baseline (%)"=w523, "Intensity Threshold"=w525, "Data In"=w532) -> ("error out"=w526:errorcluster, "Valid Fit?"=w521:bool, "Gaussian Fit Parameters"=w533:T16)  [unwired: 1 out]
          n252 = Unbundle By Name(w533) -> ("amplitude"=w529:dbl, "center"=w530:dbl, "FWHM"=w528:dbl)  [unwired: 1 out]
        }
        n253 = call <vilib>:"Add State(s) to Queue__jki_lib_state_machine.vi"("State(s) in (\"\")"=w515) -> ("States Out"=w514:string)  [unwired: 14 in]
        n254 = call-poly <userlib>:"Conditional Auto-Indexing Tunnel__ogtk.vi"("Array in"=w498, "Elements to keep"=w499) -> ("Filtered Array out"=w516:u32[])  [unwired: 5 in]
        n255 = call-poly <userlib>:"Conditional Auto-Indexing Tunnel__ogtk.vi"("Array in"=w505, "Elements to keep"=w499) -> ("Filtered Array out"=w504:dbl[])  [unwired: 5 in]
        n256 = call-poly <userlib>:"Conditional Auto-Indexing Tunnel__ogtk.vi"("Array in"=w503, "Elements to keep"=w499) -> ("Filtered Array out"=w502:dbl[])  [unwired: 5 in]
        n257 = call-poly <userlib>:"Conditional Auto-Indexing Tunnel__ogtk.vi"("Array in"=w501, "Elements to keep"=w499) -> ("Filtered Array out"=w500:dbl[])  [unwired: 5 in]
        n258 = Divide(x=w502, y=w508) -> (x/y=w511:dbl[])
        n259 = Divide(x=w500, y=w508) -> (x/y=w509:dbl[])
        n260 = in-place {
          in-place-border: w511 -> [w520]
          in-place-border: w504 -> [w519]
          in-place-border: w509 -> [w518]
          in-place-border: w516 -> [w517]
          n261 = in-place-cluster #12(w512) -> ()  [unwired: 4 out]
          n262 = in-place-cluster #12("Intensity Data.Cell Indexed.Cell Amplitude"=w519, "Intensity Data.Cell Indexed.Cell Location (um)"=w520, "Intensity Data.Cell Indexed.Cell Width (um)"=w518, "Intensity Data.Cell Indexed.Cell Location (frame)"=w517) -> (w510:T9)
        }
      }
      frame "Data Operation: Index Cell Peaks (deprecated)" {
        n263 = Unbundle By Name(w539) -> ("Intensity Data.Frame Indexed.peak location (um)"=w536:dbl[], "Gated Data.Cell Indexed.peak location (frame)"=w537:u32[])
        n264 = for {
          tunnel: w537 -> [w545] mode=indexing
          tunnel: w536 -> [w544]
          tunnel: [w543] -> w535 mode=indexing
          n265 = Index Array(array=w544, index=w545) -> (element=w543:dbl)
        }
        n266 = in-place {
          in-place-border: w535 -> [w546]
          n267 = in-place-cluster #13(w539) -> ()  [unwired: 1 out]
          n268 = in-place-cluster #13("Intensity Data.Frame Indexed.peak location (um)"=w546) -> (w538:T9)
        }
        n269 = call <vilib>:"Add State(s) to Queue__jki_lib_state_machine.vi"("State(s) in (\"\")"=w542) -> ("States Out"=w541:string)  [unwired: 14 in]
      }
      frame "Data Operation: Cell Arrival Delta - Frame" {
        n270 = Unbundle By Name(w548) -> ("Intensity Data.Cell Indexed.Cell Location (frame)"=w550:u32[])
        n271 = for {
          tunnel: w550 -> [w560] mode=indexing
          shift-right: [w560] -> _
          shift-left: _ -> [w559]
          shift-right: [w556] -> w549
          shift-left: _ -> [w558]
          i -> [w555]
          # "previous value"
          n272 = Subtract(x=w560, y=w559) -> (x-y=w557:u32)
          n273 = case "init @ 2nd iteration" shown="Default" w555 {
            tunnel: w558 -> [_ w564]
            tunnel: w557 -> [w562 w563]
            tunnel: [w561 w565] -> w556
            frame 1 {
              n274 = Build Array(w562) -> (w561:u32[])
            }
            frame Default {
              n275 = Build Array (concatenate)(w564, w563) -> (w565:u32[])
            }
          }
        }
        n276 = in-place {
          in-place-border: w549 -> [w554]
          n277 = in-place-cluster #14(w548) -> ()  [unwired: 1 out]
          n278 = in-place-cluster #14("Intensity Data.Cell Indexed.Cell Arrival Delta (frame)"=w554) -> (w547:T9)
        }
        n279 = call <vilib>:"Add State(s) to Queue__jki_lib_state_machine.vi"("State(s) in (\"\")"=w553) -> ("States Out"=w552:string)  [unwired: 14 in]
      }
      frame "Data Operation: Cell Arrival Delta - Time" {
        n280 = Unbundle By Name(w567) -> ("Intensity Data.Cell Indexed.Cell Arrival Delta (frame)"=w570:dbl[])
        n281 = Divide(x=w570, y="Frame Rate") -> (x/y=w569:dbl[])
        n282 = in-place {
          in-place-border: w569 -> [w574]
          n283 = in-place-cluster #15(w567) -> ()  [unwired: 1 out]
          n284 = in-place-cluster #15("Intensity Data.Cell Indexed.Cell Arrival Delta (us)"=w574) -> (w566:T9)
        }
        n285 = call <vilib>:"Add State(s) to Queue__jki_lib_state_machine.vi"("State(s) in (\"\")"=w573) -> ("States Out"=w572:string)  [unwired: 14 in]
      }
      frame "---------- Plot Operation ----------" {
        # "Template Separator\n(You can make a copy of, or modify, this frame)"
        n286 = call <vilib>:"Add State(s) to Queue__jki_lib_state_machine.vi"("State(s) in (\"\")"=w578) -> ("States Out"=w577:string)  [unwired: 14 in]
      }
      frame "Plot Operation: Cell Width Histogram" {
        # "Template Separator\n(You can make a copy of, or modify, this frame)"
        n287 = Unbundle By Name(w582) -> ("Intensity Data.Cell Indexed.Cell Width (um)"=w581:dbl[])
        n288 = local read "cell width histo intervals"() -> (w579:i32)
        n289 = call <vilib>:"Histogram.vi"("intervals"=w579, "X"=w581) -> ("Histogram Graph"=→"Cell Width Histogram":T3)  [unwired: 6 in, 3 out]
        n290 = call <vilib>:"Add State(s) to Queue__jki_lib_state_machine.vi"("State(s) in (\"\")"=w585) -> ("States Out"=w584:string)  [unwired: 14 in]
      }
      frame "Plot Operation: set scales for new data" {
        n291 = Unbundle By Name(w597) -> ("Intensity Data.Frame Count"=w590:u32, "Intensity Data.Pixel Count"=w588:u32)
        n292 = control-ref of="Peak Fitting"() -> (w586:refnum<vi>)
        n293 = control-ref of="Normalized Intensity Maximums"() -> (w592:refnum<vi>)
        n294 = control-ref of="Normalization Selections"() -> (w589:refnum<vi>)
        n295 = Build Array(w592, w589) -> (w591:refnum<vi>[])
        n296 = Build Array(w586) -> (w587:refnum<vi>[])
        n297 = for "plotting one frame" {
          shift-right: [w602] -> _
          shift-left: _ -> [w601]
          tunnel: w587 -> [w600] mode=indexing
          tunnel: w588 -> [w599]
          n298 = property on="Property Node" class="XYGraph (strict)"(reference=w600, error in=w601, "XScale.Maximum"=w599, "XScale.Minimum"=0.0 ("X Scale.Range:Minimum")) -> (error out=w602:errorcluster)  [unwired: 1 out]
        }
        n299 = for "plotting all frames" {
          shift-right: [w607] -> w593
          shift-left: w596 -> [w606]
          tunnel: w591 -> [w605] mode=indexing
          tunnel: w590 -> [w604]
          n300 = property on="Property Node" class="XYGraph"(reference=w605, error in=w606, "XScale.Maximum"=w604, "XScale.Minimum"=0.0 ("X Scale.Range:Minimum")) -> (error out=w607:errorcluster)  [unwired: 1 out]
        }
        n301 = call <vilib>:"Add State(s) to Queue__jki_lib_state_machine.vi"("State(s) in (\"\")"=w595) -> ("States Out"=w594:string)  [unwired: 14 in]
      }
      frame "Plot Operation: plot raw data" {
        n302 = Unbundle By Name(w612) -> ("Intensity Data.Raw Data"=w609:i32[][])
        n303 = for {
          tunnel: [w618] -> w611 mode=indexing
          tunnel: w609 -> [w617] mode=indexing
          tunnel: [w616] -> w608 mode=indexing
          i -> [w618]
          n304 = Array Max & Min(array=w617) -> (max value=w616:i32)  [unwired: 3 out]
        }
        n305 = Bundle(w611, w608) -> (→"Normalization Selections":cluster{i32[], i32[]})  [unwired: 1 in]
        n306 = call <vilib>:"Add State(s) to Queue__jki_lib_state_machine.vi"("State(s) in (\"\")"=w615) -> ("States Out"=w614:string)  [unwired: 14 in]
      }
      frame "Plot Operation: plot cell locations" {
        # "cell peak locations"
        # "intensity data"
        n307 = Unbundle By Name(w629) -> ("Intensity Data.Cell Indexed.Cell Location (frame)"=w620:u32[], "Intensity Data.Cell Indexed.Cell Amplitude"=w628:dbl[], "Intensity Data.Frame Indexed.intensity peak"=w623:dbl[])
        n308 = Array Size(array=w623) -> (size(s)=w627:i32)
        n309 = Array Size(array=w620) -> (size(s)=w619:i32)
        n310 = for {
          N: w627 -> [_]
          tunnel: [w632] -> w626 mode=indexing
          i -> [w632]
        }
        n311 = local write "Cells Identified"(w619) -> ()
        n312 = Bundle("Cell Location (frame)"=w620, "Cell Amplitude"=w628) -> (w624:T17)  [unwired: 1 in]
        n313 = Bundle(w626, "intensity peak"=w623) -> (w622:cluster{i32[], "intensity peak":dbl[]})  [unwired: 1 in]
        n314 = Build Array(w622, w624) -> (→"Normalized Intensity Maximums":T2)
        n315 = call <vilib>:"Add State(s) to Queue__jki_lib_state_machine.vi"("State(s) in (\"\")"=w631) -> ("States Out"=w630:string)  [unwired: 14 in]
      }
      frame "Plot Operation: initialize fitting plot" {
        w633 = u32 10 ("element")
        n316 = Unbundle By Name(w636) -> ("Intensity Data.Pixel Count"=w635:u32)
        n317 = property on="Peak Fitting" class="XYGraph (strict)"() -> ("CrsrList"=w644:T11)  [unwired: 2 in, 2 out]
        n318 = Index Array(array=w644) -> (element #1=w643:T12, element #2=w642:T12)  [unwired: 2 in]
        n319 = Subtract(x=w635, y=w633) -> (x-y=w634:u32)
        n320 = in-place {
          in-place-border: w633 -> [w649]
          in-place-border: w634 -> [w648]
          n321 = in-place-cluster #16(w643) -> ()  [unwired: 1 out]
          n322 = in-place-cluster #17(w642) -> ()  [unwired: 1 out]
          n323 = in-place-cluster #16("Position.X"=w649) -> (w641:T12)
          n324 = in-place-cluster #17("Position.X"=w648) -> (w640:T12)
        }
        n325 = Build Array(w641, w640) -> (w639:T13)
        n326 = Build Array(w633, w634) -> (w638:u32[])
        n327 = property on="Peak Fitting" class="XYGraph (strict)"("CrsrList"=w639) -> ()  [unwired: 2 in, 2 out]
        n328 = Bundle By Name(cluster=w636, "Intensity Data.Fitting Range"=w638) -> (w637:T9)
        n329 = call <vilib>:"Add State(s) to Queue__jki_lib_state_machine.vi"("State(s) in (\"\")"=w647) -> ("States Out"=w646:string)  [unwired: 14 in]
      }
      frame "Plot Operation: Plot Cell Arrival Histogram" {
        n330 = Unbundle By Name(w661) -> ("Intensity Data.Cell Indexed.Cell Arrival Delta (us)"=w652:dbl[])
        n331 = local read "delta threshold"() -> (w655:dbl)
        n332 = Sort 1D Array(array=w652) -> (sorted array=w650:dbl[])
        n333 = Threshold 1D Array(2:w655, 3:w650) -> (0:w654:dbl)  [unwired: 1 in]
        n334 = Round Toward +Infinity(x=w654) -> (ceil(x): smallest int >= x=w653:dbl)
        n335 = Array Subset(array=w650, index=w653) -> (w651:dbl[])  [unwired: 1 in]
        n336 = call <vilib>:"Histogram.vi"("intervals"="arrival histogram interval", "X"=w651) -> ("error"=w658:i32, "Histogram Graph"=→"Arrival time delta histogram":T3)  [unwired: 6 in, 2 out]
        n337 = call <vilib>:"Add State(s) to Queue__jki_lib_state_machine.vi"("State(s) in (\"\")"=w663) -> ("States Out"=w662:string)  [unwired: 14 in]
        n338 = call <vilib>:"Error Cluster From Error Code.vi"("error in (no error)"=w657, "error code (0)"=w658) -> ("error out"=w656:errorcluster)  [unwired: 7 in]
      }
      frame "Plot Operation: Plot Selected Frame" {
        n339 = Unbundle By Name(w679) -> ("Intensity Data.Normalized Intensity Data"=w676:dbl[][])
        n340 = property on="Normalized Intensity Maximums" class="XYGraph (strict)"(error in=w678) -> (error out=w668:errorcluster, "Cursor.Cursor X"=w677:dbl)  [unwired: 1 in, 1 out]
        "Selected Frame" <- w677
        n341 = Index Array "grab frame"(array=w676, index (row)=w677) -> (element=w670:dbl[])  [unwired: 1 in]
        n342 = local read "Gaussian Fit Method"() -> (w682:T1)
        n343 = local read "Intensity Threshold"() -> (w669:i32)
        n344 = local read "Target Baseline (%)"() -> (w665:dbl)
        n345 = local read "Padding"() -> (w664:u32)
        n346 = call <vilib>:"Add State(s) to Queue__jki_lib_state_machine.vi"("State(s) in (\"\")"=w681) -> ("States Out"=w680:string)  [unwired: 14 in]
        n347 = call "Find Intensity Peaks V3.vi"("Gaussian Fit Method"=w682, "Padding"=w664, "error in (no error)"=w668, "Target Baseline (%)"=w665, "Intensity Threshold"=w669, "Data In"=w670) -> ("error out"=w667:errorcluster, "Gaussian Fit Parameters"=w675:T16, "All Data (X,Y)"=→"Peak Fitting":cluster{"Locations":dbl[], "Amplitudes":dbl[]}[])  [unwired: 1 out]
        n348 = Unbundle By Name(w675) -> ("amplitude"=→"amplitude":dbl, "center"=→"center":dbl, "FWHM"=→"FWHM":dbl, "residue"=→"residue":dbl)
      }
      frame "Plot Operation: Draw Histogram" {
        # "um location of peaks"
        # "Template Separator\n(You can make a copy of, or modify, this frame)"
        n349 = Unbundle By Name(w688) -> ("Intensity Data.Cell Indexed.Cell Location (um)"=w683:dbl[])
        n350 = local read "location histogram interval"() -> (w689:i32)
        n351 = Array Size(array=w683) -> (size(s)=→"Cell Count":i32)
        n352 = call <vilib>:"Histogram.vi"("intervals"=w689, "X"=w683) -> ("error"=w687:i32, "Histogram Graph"=→"Cell Location histogram":T3)  [unwired: 6 in, 2 out]
        n353 = call <vilib>:"Add State(s) to Queue__jki_lib_state_machine.vi"("State(s) in (\"\")"=w692) -> ("States Out"=w691:string)  [unwired: 14 in]
        n354 = call <vilib>:"Error Cluster From Error Code.vi"("error in (no error)"=w686, "error code (0)"=w687) -> ("error out"=w685:errorcluster)  [unwired: 7 in]
      }
      frame "Plot Operation: Micron Range" {
        # "Template Separator\n(You can make a copy of, or modify, this frame)"
        n355 = Unbundle By Name(w698) -> ("Intensity Data.Interrogation Width (um)"=w693:dbl)
        n356 = control-ref of="Cell Location histogram"() -> (w697:refnum<vi>)
        n357 = property on="Property Node" class="XYGraph (strict)"(reference=w697, error in=w702, "XScale.Maximum"=w693, "XScale.Minimum"=0.0 ("X Scale.Range:Minimum")) -> (reference out=w696:refnum<vi>, error out=w695:errorcluster)
        n358 = Close Reference(reference=w696, error in (no error)=w695) -> (error out=w694:errorcluster)
        n359 = call <vilib>:"Add State(s) to Queue__jki_lib_state_machine.vi"("State(s) in (\"\")"=w701) -> ("States Out"=w700:string)  [unwired: 14 in]
      }
      frame "---------- Statistics ----------" {
        # "Template Separator\n(You can make a copy of, or modify, this frame)"
        n360 = call <vilib>:"Add State(s) to Queue__jki_lib_state_machine.vi"("State(s) in (\"\")"=w706) -> ("States Out"=w705:string)  [unwired: 14 in]
      }
      frame "Statistics: Gate Population" {
        n361 = Unbundle By Name(w724) -> ("Intensity Data.Cell Indexed.Cell Location (um)"=w718:dbl[], "Gated Data.Gate Center"=w721:u32, "Gated Data.Gate Width"=w720:u32, "Intensity Data.Cell Indexed.Cell Amplitude"=w716:dbl[], "Intensity Data.Cell Indexed.Cell Location (frame)"=w715:u32[])
        n362 = call "Gate Data.vi"("Data In"=w718, "Gate Center"=w721, "Gate Width"=w720) -> ("Gated Data Out"=w722:dbl[], "Indeces Used"=w717:i32[], "% population in gate"=→"% population\nin gate":dbl, "Gate Position (min,max)"=w710:dbl[])
        n363 = Index Array(array=w710) -> (element #1=w709:dbl, element #2=w708:dbl)  [unwired: 2 in]
        n364 = call-poly <userlib>:"Index Array Elements__ogtk.vi"("indices"=w717, "array"=w716) -> ("elements"=w714:dbl[])  [unwired: 9 in]
        n365 = call-poly <userlib>:"Index Array Elements__ogtk.vi"("indices"=w717, "array"=w715) -> ("elements"=w713:u32[])  [unwired: 9 in]
        n366 = in-place {
          in-place-border: w722 -> [w729]
          in-place-border: w714 -> [w728]
          in-place-border: w713 -> [w727]
          n367 = in-place-cluster #18(w724) -> ()  [unwired: 3 out]
          n368 = in-place-cluster #18("Gated Data.Cell Indexed.peak location (um)"=w729, "Gated Data.Cell Indexed.Peak Amplitude"=w728, "Gated Data.Cell Indexed.peak location (frame)"=w727) -> (w723:T9)
        }
        n369 = control-ref of="Cell Location histogram"() -> (w707:refnum<vi>)
        n370 = call "Draw Gate.vi"("error in (no error)"=w712, "Upper Limit"=w708, "Lower Limit"=w709, "XYGraph reference"=w707) -> ("error out"=w711:errorcluster)  [unwired: 3 in]
        n371 = call <vilib>:"Add State(s) to Queue__jki_lib_state_machine.vi"("State(s) in (\"\")"=w726) -> ("States Out"=w725:string)  [unwired: 14 in]
      }
      frame "Statistics: Find Best Gate Center" {
        n372 = Unbundle By Name(w732) -> ("Intensity Data.Interrogation Width (um)"=w734:dbl, "Intensity Data.Cell Indexed.Cell Location (um)"=w738:dbl[], "Gated Data.Gate Width"=w739:u32)
        n373 = Round Toward +Infinity(x=w734) -> (ceil(x): smallest int >= x=w733:dbl)
        n374 = for {
          N: w733 -> [_]
          tunnel: w739 -> [w747]
          tunnel: w738 -> [w746]
          tunnel: [w745] -> w735 mode=indexing
          tunnel: [w744] -> w737 mode=indexing
          i -> [w745]
          n375 = call "Gate Data.vi"("Data In"=w746, "Gate Center"=w745, "Gate Width"=w747) -> ("% population in gate"=w744:dbl)  [unwired: 3 out]
        }
        n376 = Array Max & Min(array=w737) -> (max index (indices)=w736:i32)  [unwired: 3 out]
        n377 = Index Array(array=w735, index=w736) -> (element=w730:i32)
        n378 = in-place {
          in-place-border: w730 -> [w743]
          n379 = in-place-cluster #19(w732) -> ()  [unwired: 1 out]
          n380 = in-place-cluster #19("Gated Data.Gate Center"=w743) -> (w731:T9)
        }
        n381 = local write "Gate Center"(w730) -> ()
        n382 = call <vilib>:"Add State(s) to Queue__jki_lib_state_machine.vi"("State(s) in (\"\")"=w742) -> ("States Out"=w741:string)  [unwired: 14 in]
      }
      frame "---------- File Operation ----------" {
        # "Template Separator\n(You can make a copy of, or modify, this frame)"
        n383 = call <vilib>:"Add State(s) to Queue__jki_lib_state_machine.vi"("State(s) in (\"\")"=w751) -> ("States Out"=w750:string)  [unwired: 14 in]
      }
      frame "File Operation: Choose Data Set" {
        # "canceled?"
        # "Template Separator\n(You can make a copy of, or modify, this frame)"
        n384 = case "2D array?" shown="True" "Array Type" {
          tunnel: w761 -> [w765 w771]
          tunnel: [w764 w770] -> w760
          tunnel: [w763 w769] -> w755
          tunnel: [w762 w767] -> w753
          frame False {
            n385 = call "File Dialog"("prompt"="Choose folder with intensity data. Code will analyze ALL .txt files!", "error in"=w765) -> ("selected path"=w762:path, "cancelled"=w763:bool, "error out"=w764:errorcluster)  [unwired: 10 in, 1 out]
          }
          frame True {
            n386 = call "File Dialog2"("prompt"="Choose file", "error in"=w771) -> ("selected path"=w767:path, "cancelled"=w769:bool, "error out"=w770:errorcluster)  [unwired: 10 in, 1 out]
          }
        }
        n387 = in-place {
          in-place-border: w755 -> [w775]
          in-place-border: w753 -> [w772]
          n388 = in-place-cluster #20(w759) -> ("Intensity Data Location"=w774:path)
          n389 = Select(t=w774, s=w775, f=w772) -> (s? t:f=w773:path)
          n390 = in-place-cluster #20("Intensity Data Location"=w773) -> (w758:T9)
        }
        n391 = Select(t="", s=w755, f=w757) -> (s? t:f=w756:string)
      }
      frame "File Operation: Import Data" {
        # "row = frame #\ncolumn = pixel #"
        # "um/pixels"
        n392 = Unbundle By Name(w785) -> ("pixels/um"=w783:dbl, "Intensity Data Location"=w788:path)
        n393 = local read "Array Type"() -> (w780:bool)
        n394 = Reciprocal(x=w783) -> (1/x=w782:dbl)
        n395 = case shown="True" w780 {
          tunnel: w788 -> [w794 w798]
          tunnel: w787 -> [w793 w799]
          tunnel: [w792 w799] -> w786
          tunnel: [w791 w796] -> w779
          frame False {
            n396 = call "Read all txt files to numeric array.vi"("error in (no error)"=w793, "selected folder"=w794) -> ("error out"=w792:errorcluster, "Data Out"=w791:i32[][])  [unwired: 1 in, 1 out]
          }
          frame True {
            n397 = call-poly <vilib>:"Read From Spreadsheet File.vi"("transpose (no:F)"=TRUE, "file path (dialog if empty)"=w798) -> ("all rows"=w797:i64[][])  [unwired: 5 in, 4 out]
            n398 = To Long Integer(number=w797) -> (32bit integer=w796:i32[][])
          }
        }
        n399 = Array Size(array=w779) -> (size(s)=w778:i32[])
        n400 = Index Array(array=w778) -> (element #1=w777:i32, element #2=w776:i32)  [unwired: 2 in]
        n401 = Multiply(x=w782, y=w776) -> (x*y=w781:dbl)
        n402 = in-place {
          in-place-border: w779 -> [w803]
          in-place-border: w781 -> [w802]
          in-place-border: w776 -> [w801]
          in-place-border: w777 -> [w800]
          n403 = in-place-cluster #21(w785) -> ()  [unwired: 4 out]
          n404 = in-place-cluster #21("Intensity Data.Raw Data"=w803, "Intensity Data.Frame Count"=w800, "Intensity Data.Pixel Count"=w801, "Intensity Data.Interrogation Width (um)"=w802) -> (w784:T9)
        }
        n405 = call <vilib>:"Add State(s) to Queue__jki_lib_state_machine.vi"("State(s) in (\"\")"=w790) -> ("States Out"=w789:string)  [unwired: 14 in]
      }
    }
  }
  n406 = call <vilib>:"Add State(s) to Queue__jki_lib_state_machine.vi"() -> ()  [unwired: 15 in, 1 out]
